vi "Preference_Panel.vi"(0 "Mode":T2) -> ()   [LabVIEW 2012]
uses:
  Anemometry Sub Vis/Controls/Server_Comms.ctl
  Anemometry Sub Vis/Controls/Preference_Mode.ctl
  Anemometry Sub Vis/Controls/EnFlo_Data_Folder_Setup.ctl
  Anemometry Sub Vis/File/Setup_Filetype.ctl
  Anemometry Sub Vis/Controls/Overhead.ctl
  <vilib>/Instr/_visa.llb/VISA Find Search Mode.ctl
  ADAM Client/Sub VIs/ADAM Controls/Ch_description_ADAM.ctl
  ADAM Client/Sub VIs/ADAM Controls/Module_type_ADAM.ctl
  ADAM Client/Sub VIs/ADAM Controls/Function_ADAM.ctl
  ADAM Client/Sub VIs/ADAM Controls/Channel_State.ctl
  ADAM Client/Sub VIs/ADAM Controls/Calib_type_ADAM.ctl
  ADAM Client/Sub VIs/ADAM Controls/Address.ctl
  Anemometry Sub Vis/Globals/Constants_global.vi
  Anemometry Sub Vis/Globals/Preference_global.vi
  Anemometry Sub Vis/Globals/Trav_pos_global.vi
  Anemometry Sub Vis/Acquisition/PWA/PWAtasksGLOBAL.vi
panel:
  in  "Traverse to Traverse Collision Detection":bool
  in  "DataTranslation Device No.":u32=20
  in  "Reset Email Counter":bool
  in  "EnFlo_Data_Folder_Setup":T1="EnFlo_Data on Server"
  in  "Post Processing Machine":bool
  in  "Analogue Device Serial No.":string="1188AB4"
  in  "PWA Device Serial No.":string="1187C98"
  in  "ADAM Setup File":u16(ring) items=["Scani_Valve.xls", "Current_Setup.xls"]
  in  "Default Source Establishment Time (s)":dbl=20.0
  out "This Machine's IP Number":string
  in  "Rig Setup":u16(ring) items=["3_x_2_tunnel", "A_Tunnel", "Adam_Sayer_Desk", "ADAM_Server", "Aero_Tunnel", "Alex_Desktop", "B_Tunnel", "Calibration_Tunnel", "Contact_Conductance", "D_Tunnel", "EnFlo_Tunnel", "Frauke_Desktop", "Fruit_Rig", "iMac_G5_2", "iMacDuo1", "Matteo's_desktop", "Matteo_PC", "Nick_PC-2", "Paul_Desk-Paul_Desk_Machine", "Paul_Hayden-Desk", "Paul_N_Desk_Machine_2", "phtest", "Post_Processing_Machine", "PowerBook_G4_1", "PowerBook_G4_2", "Syn_jet_rig", "Tank", "tdf", "Tom_Desk", "Towing_tank", "--New Rig Setup--"]
  in  "Default Traverse Name":u16(ring) items=["A_Tunnel", "Aero_Laser", "Aero_ThroughWall", "Aero_Tunnel", "Angle_Calibrator", "B_Tunnel", "D_Tunnel", "Dummy_Traverse", "EnFlo_Stack", "EnFlo_Tunnel", "EnFlo_Turntable", "Laser_Meas_Traverse", "mohd_setup", "Paul_Desk_Test", "PIV_Traverse", "--New Traverse Setup--"]
  in  "OK":bool
  in  "% Error From First Calib":dbl=10.0 format="%.1f"
  in  "% Error From Previous Calib":dbl=0.5 format="%.1f"
  out "Templates":path=path "/G4_2_HD/Applications (Mac OS 9)/EnFlo Software/Anemometry/Anemometry Sub Vis/Templates"
  in  "Data Folder":path
  out "EnFlo SW Preferences":path=path "/G4_2_HD/Applications (Mac OS 9)/LabVIEW 5.1/EnFlo SW Preferences"
  in  "Tunnel Speed Control":bool
  in  "SMTP server IP address":string
  in  "Abs Press (mbar)":string="Froude:NPL:Atmos_Press"
  in  "Temperature":string="EnFlo Tun:Inlet Heater:Av Temp"
  in  "Server port number":u32=3363
  in  "Server address":string
  in  "LabVIEW Administrators":string[](array[string])=["", "", "", "", "", "", "", "", "", "", "", "", "", "", "", "", "", "", "", ""]
  in  "Server Comms":T3=enum."Do Not Link To Server"
  # "Server Computer Peferences"
  # "Multi Run Preferences"
  # "Warning Levels for Autocalibration Changes"
  # "Email Peferences"
  # "Deg C"
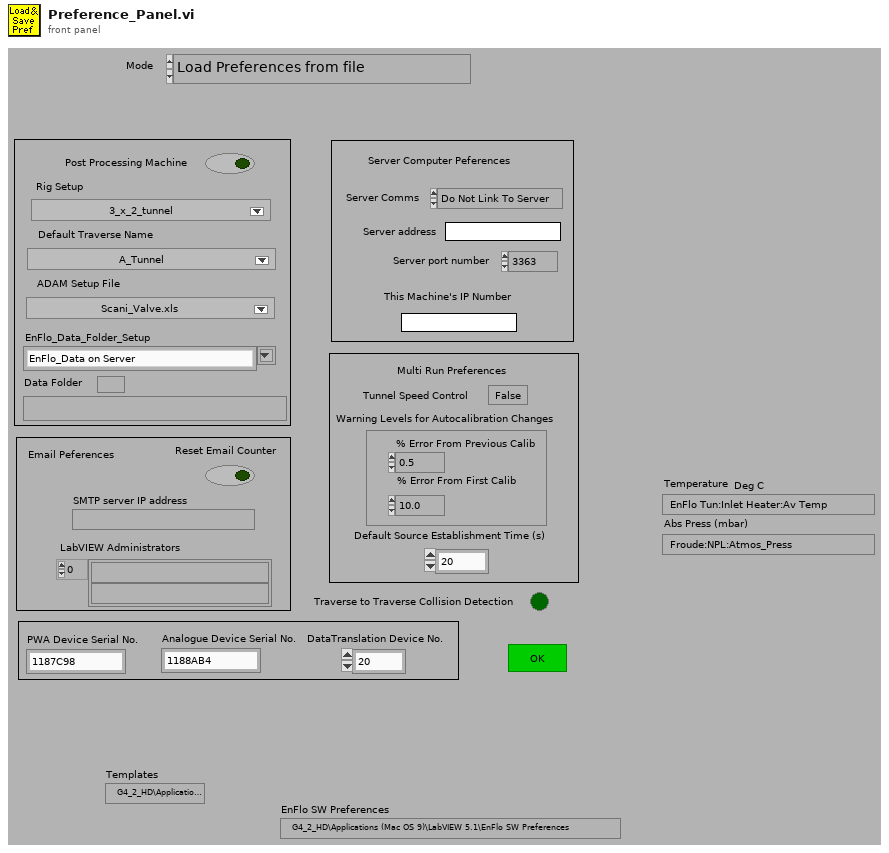
[diagram p1: front panel]
types:
  T1 = typedef "EnFlo_Data_Folder_Setup.ctl" = string
  T2 = typedef "Preference_Mode.ctl" = enum16{"Load Preferences from file", "Save Preferences to file", "Load, Edit then Save"}
  T3 = typedef "Server_Comms.ctl" = enum16{"Server Link Healthy", "Do Not Link To Server"}
  T4 = enum8{"Enabled", "Disabled", "Disabled and Grayed Out"}
  T5 = enum16{"Zero or one", "One", "Zero or more", "One or more"}
  T6 = typedef "Setup_Filetype.ctl" = enum16{"Measurement Setups", "Calibration Setups", "General", "Results File Plotter Setups", "Speed Calib Tweaks"}
  T7 = typedef "Overhead.ctl" = enum16{"Update total times", "Read Current Overhead", "Re Scale totals to 3 hrs", "Initialise totals to 3hr"}
  T8 = typedef "Calib_type_ADAM.ctl" = enum16{"Raw", "Bx + A", "Cx^2 + Bx + A", "Dx^3 + Cx^2 + Bx + A", "In Band", "Hi-Tec Q", "Hi-Tec M_dot", "Text"}
  T9 = typedef "Module_type_ADAM.ctl" = string
  T10 = typedef "Channel_State.ctl" = enum16{"On", "Off", "Always On", "Always Off"}
  T11 = typedef "LVDateTimeRec.ctl" = cluster{"fractional second":dbl, "second":i32, "minute":i32, "hour":i32, "day of month":i32, "month":i32, "year":i32, "day of week":i32, "day of year":i32, "DST":i32}
  T12 = typedef "VISA Find Search Mode.ctl" = u32
  T13 = typedef "Ch_description_ADAM.ctl" = cluster{"Ch Name":string, "Type":T9, "Function":T14, "Ch State":T10, "Calibration type":T8, "A":dbl, "B":dbl, "C":dbl, "D":dbl, "Comments":string, "Address":T15, "String":string, "Duty":u16}
  T14 = typedef "Function_ADAM.ctl" = enum16{"Analogue Input", "Digital Input", "Event counter", "Event rate", "Analogue Output", "Digital Output", "Relay Output"}
  T15 = typedef "Address.ctl" = cluster{"Main":i32, "Ch.":i32, "Sub":i32, "Port Name":string}
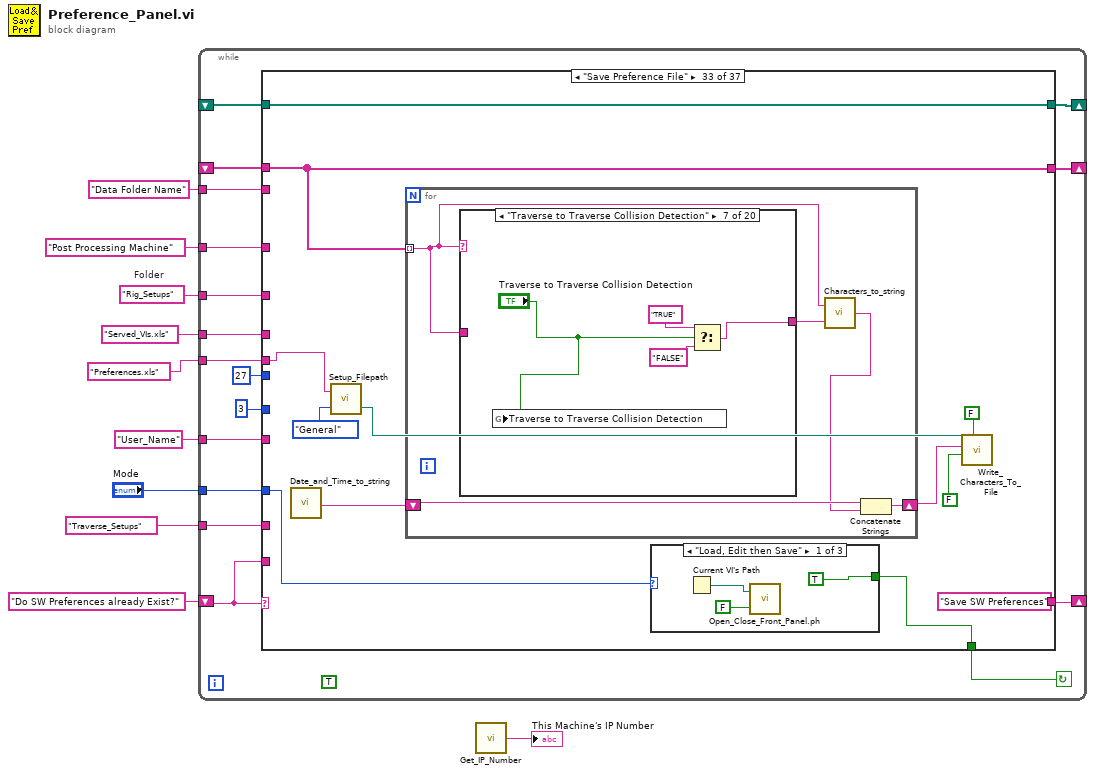
[diagram p0: block diagram]
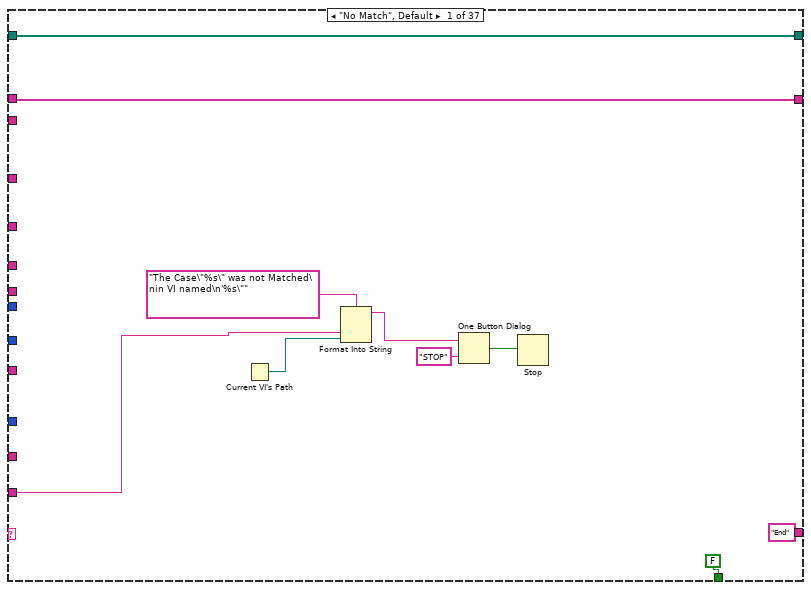
[diagram p2: hidden frame]
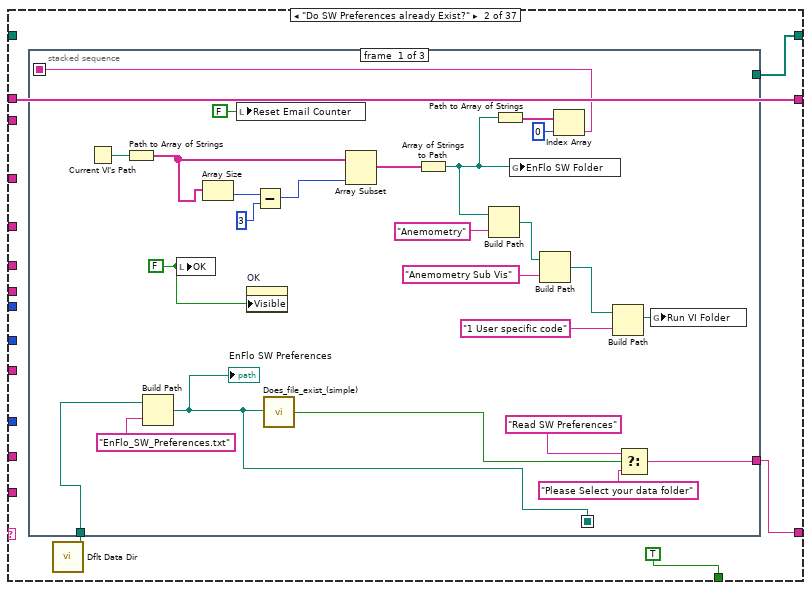
[diagram p3: hidden frame]
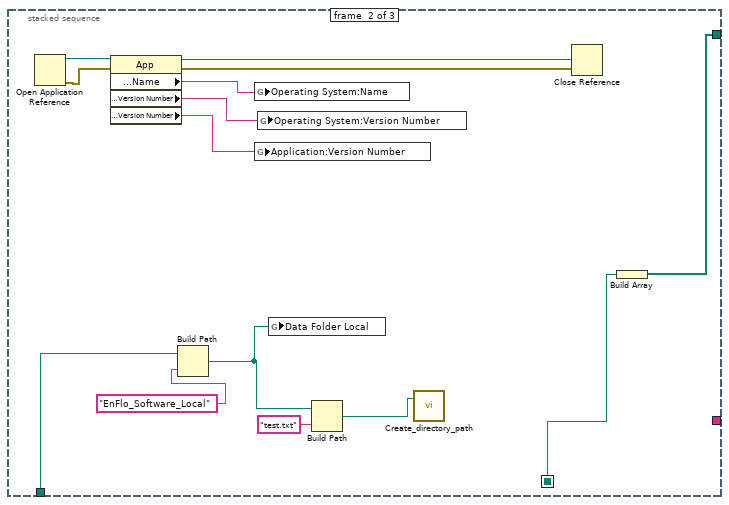
[diagram p4: hidden frame]
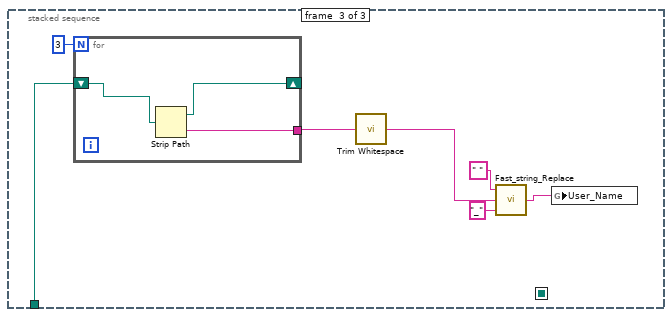
[diagram p5: hidden frame]
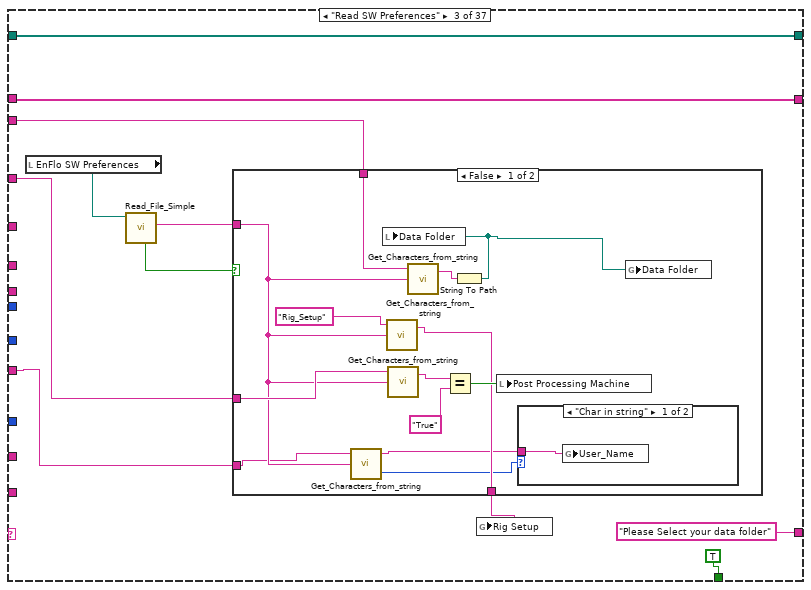
[diagram p6: hidden frame]
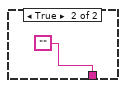
[diagram p8: hidden frame]
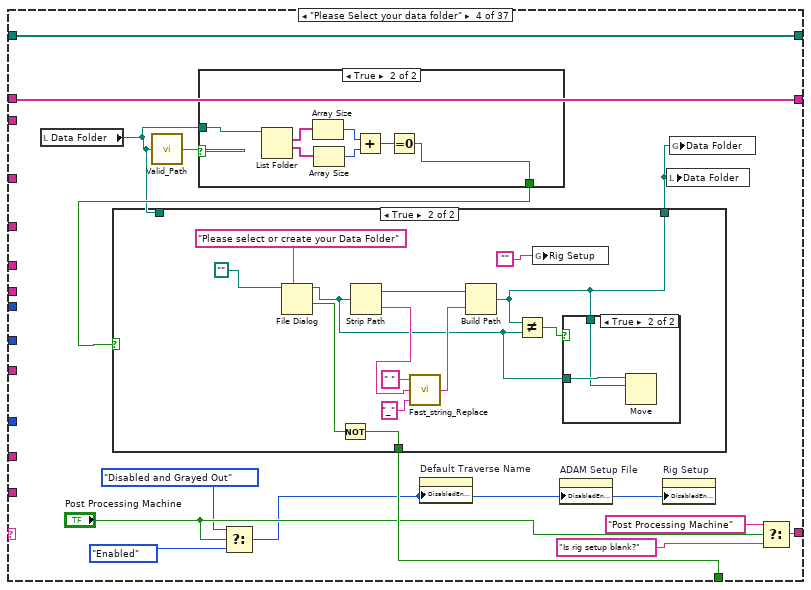
[diagram p9: hidden frame]
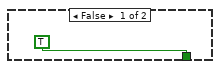
[diagram p10: hidden frame]
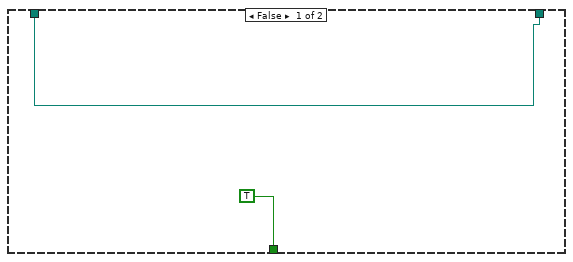
[diagram p11: hidden frame]
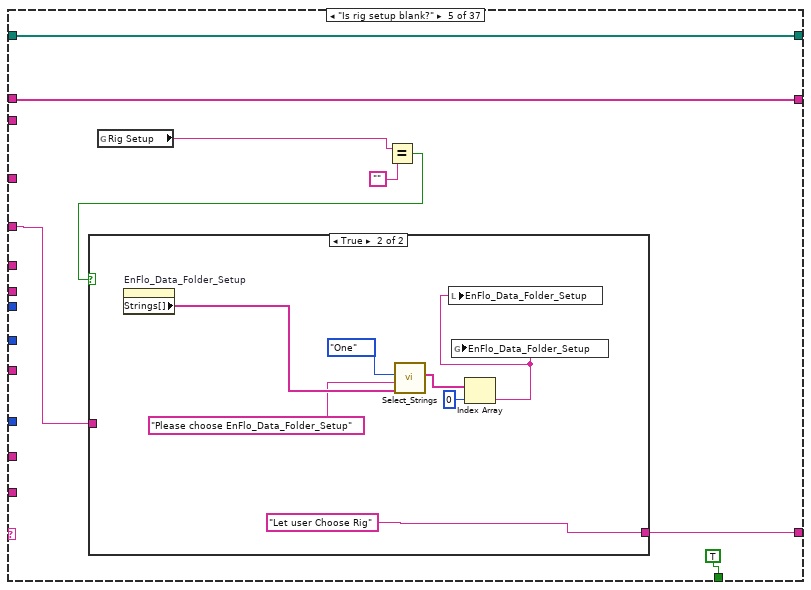
[diagram p13: hidden frame]
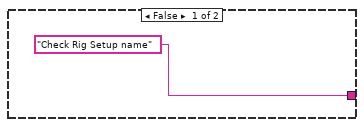
[diagram p14: hidden frame]
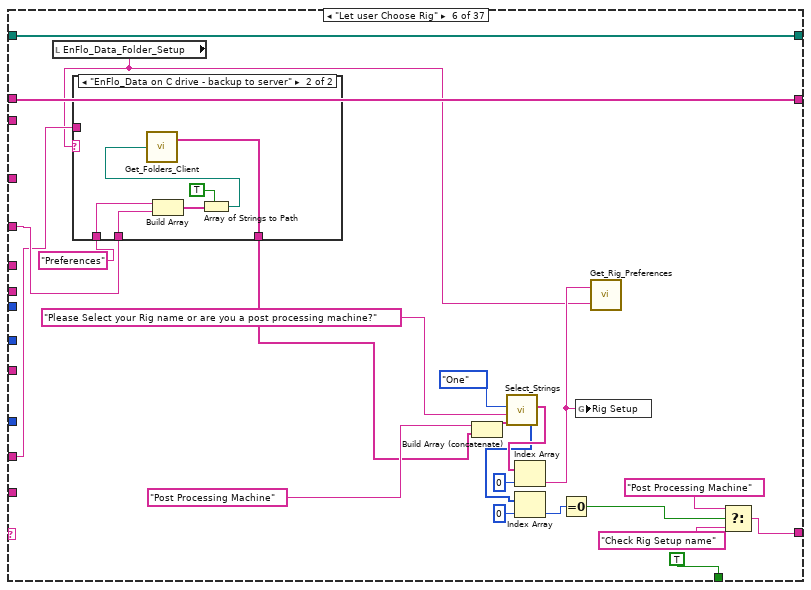
[diagram p15: hidden frame]
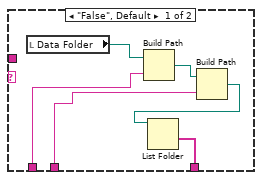
[diagram p16: hidden frame]
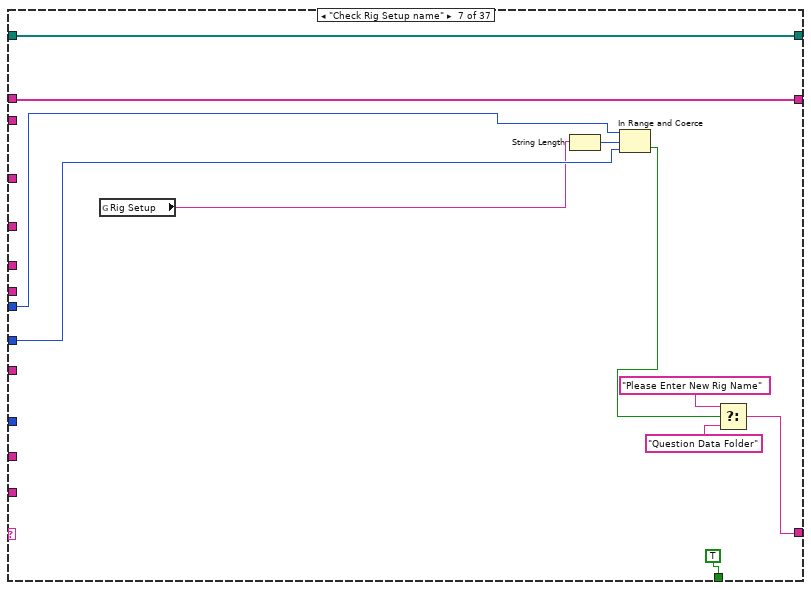
[diagram p17: hidden frame]
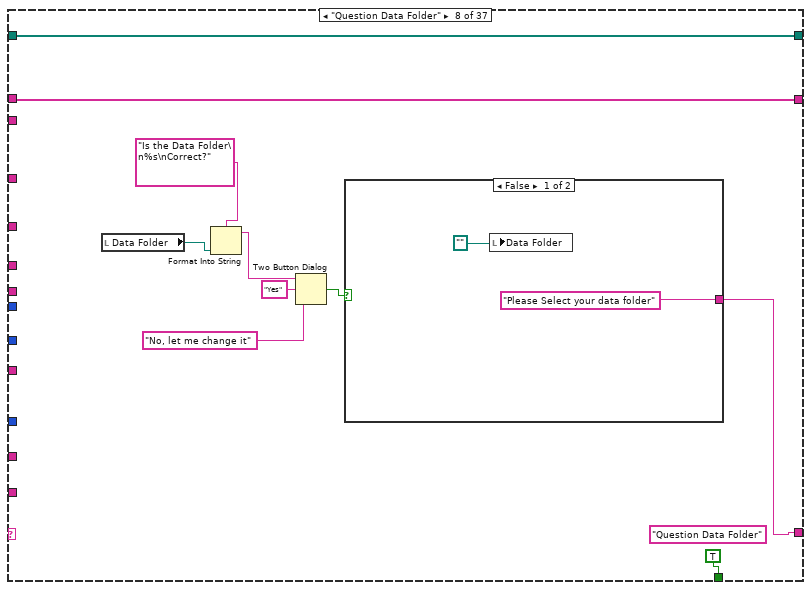
[diagram p18: hidden frame]
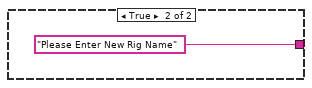
[diagram p19: hidden frame]
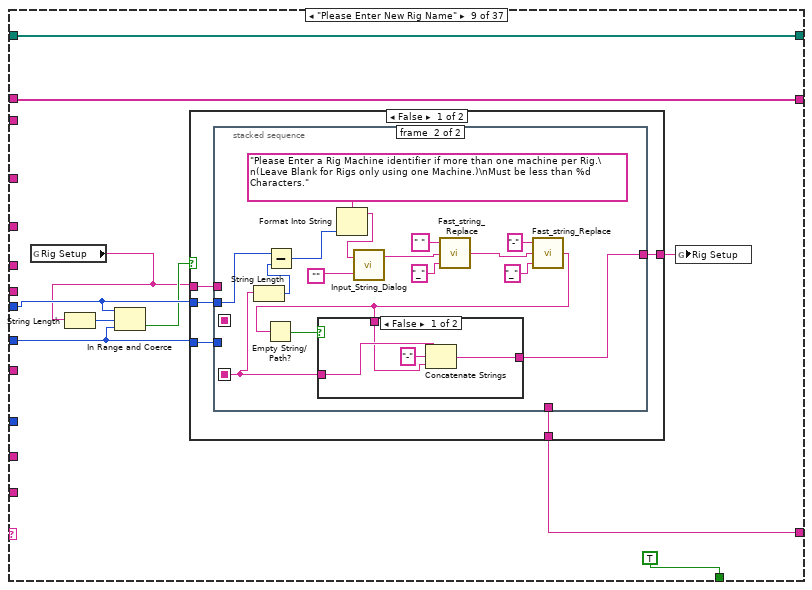
[diagram p20: hidden frame]
diagram:
  w5 = "Rig_Setups"  # Folder
  n1 = while {
    shift-left: _ -> [w24]
    shift-right: [w25] -> _
    shift-left: "Do SW Preferences already Exist?" -> [w12]
    shift-right: [w26] -> _
    tunnel: "Mode" -> [w23]
    tunnel: "Data Folder Name" ("Label for characters") -> [w22]
    tunnel: "Served_VIs.xls" ("Substring") -> [w21]
    tunnel: "Preferences.xls" ("name or relative path") -> [w20]
    tunnel: w5 -> [w17]
    tunnel: "Traverse_Setups" ("name or relative path") -> [w16]
    shift-right: [w15] -> _
    shift-left: _ -> [w14]
    tunnel: "Post Processing Machine" ("Label for characters") -> [w13]
    tunnel: "User_Name" ("Label for characters") -> [w11]
    stop <- w27 continue-if-true
    (unwired) TRUE ("append to file? (new file:F)")
    n2 = case shown="\"Save Preference File\"" w12 {
      tunnel: [FALSE TRUE TRUE w125 TRUE TRUE TRUE TRUE TRUE TRUE TRUE TRUE TRUE TRUE TRUE TRUE TRUE TRUE TRUE TRUE TRUE TRUE TRUE TRUE TRUE TRUE TRUE TRUE TRUE TRUE TRUE TRUE w924 TRUE TRUE TRUE FALSE] -> w27
      tunnel: ["End" w40 "Please Select your data folder" w122 w157 w190 w207 w218 w237 "Update Constants Global" ("f") "Copy Preferences?" "Copy Preferences?" w365 w375 "Install Preference files" "Install Adam table files" "Install Adam setup files" "Choose ADAM Setup file" "Preference files continued" "Variable Names" w553 w573 "Please Enter new  Traverse Setup" w652 "Create Traverse setup" ("f") "Check file permission status" w749 w780 w800 w820 w836 "Save Preference File" "Save SW Preferences" w999 w1013 "Initialise Globals" "End"] -> w26
      tunnel: [w29 w41 w101 w131 w163 w193 w216 w226 w239 w304 w330 w353 w363 w380 w438 w453 w478 w497 w519 w529 w558 w580 w640 w654 w688 w705 w750 w785 w805 w828 w841 w855 w930 w1007 w1014 w1066 w1125] -> w25
      tunnel: w24 -> [w29 w41 w101 w131 w163 w193 w216 w226 w239 w304 w330 w353 w363 w380 w438 w453 w478 w497 w519 w529 _ w580 w640 w654 w688 w705 w750 w785 w805 w828 w841 w855 w930 w1007 w1014 w1066 w1125]
      tunnel: w12 -> [w32 _ _ _ _ _ _ _ _ _ _ _ _ _ _ _ _ _ _ _ _ _ _ _ _ _ _ _ _ _ _ _ _ _ _ _ _]
      tunnel: w23 -> [_ _ _ _ _ _ _ _ _ _ _ _ _ _ _ _ _ _ _ _ w552 _ _ _ _ _ w748 _ _ _ _ _ w925 _ _ _ _]
      tunnel: w22 -> [_ _ w98 _ _ _ _ _ _ _ _ _ _ _ _ _ _ _ _ _ _ _ _ _ _ _ _ _ _ _ _ _ _ w998 _ _ _]
      tunnel: w21 -> [_ _ _ _ _ _ _ _ _ _ _ _ _ _ _ w448 _ _ _ _ _ _ _ _ _ _ _ _ _ _ _ _ _ _ _ w1058 _]
      tunnel: w20 -> [_ _ _ _ _ _ _ _ _ _ _ _ w359 w379 _ _ _ _ _ _ _ w570 _ _ _ _ _ _ _ _ _ _ w921 _ _ _ _]
      tunnel: 3 ("lower limit") -> [_ _ _ _ _ _ w212 _ w236 _ _ _ _ _ _ _ _ _ _ _ _ _ _ w651 _ _ _ _ _ _ _ _ _ _ _ _ _]
      tunnel: 27 ("upper limit") -> [_ _ _ _ _ _ w213 _ w235 _ _ _ _ _ _ _ _ _ _ _ _ _ _ w650 _ _ _ _ _ _ _ _ _ _ _ _ _]
      tunnel: w17 -> [_ _ _ _ w160 w178 _ _ _ w292 w318 _ _ w378 _ _ _ _ _ _ _ _ _ _ _ _ _ _ _ _ _ _ _ _ _ _ _]
      tunnel: w16 -> [_ _ _ _ _ w175 _ _ _ _ _ _ _ _ _ _ _ _ _ _ _ _ w638 _ w675 _ _ _ _ _ _ w854 _ _ _ _ _]
      tunnel: [w28 w38 w97 w126 w158 w192 w215 w225 w231 w290 w315 w342 w364 w381 w431 w444 w471 w494 w505 w521 w545 w576 w637 w646 w674 w701 path[] [] w777 w797 w823 w839 w853 w923 w995 w1012 w1060 w1123] -> w15
      tunnel: w14 -> [w28 _ w97 w126 w158 w192 w215 w225 w231 w290 w315 w342 w364 w381 w430 w446 w471 w495 w505 w523 w545 w577 w637 w646 w674 w702 w747 w777 w797 w823 w839 w853 w923 w995 w1012 w1060 w1123]
      tunnel: w13 -> [_ _ w96 _ _ _ _ _ _ _ _ _ _ _ _ _ _ _ _ _ _ _ _ _ _ _ _ _ _ _ _ _ _ w989 _ _ _]
      tunnel: w11 -> [_ _ w92 _ _ _ _ _ _ _ _ _ _ _ _ _ _ _ _ _ _ _ _ _ _ _ _ _ _ _ _ _ _ w988 _ _ _]
      frame "No Match", Default {
        n3 = Current VI's Path() -> (path=w37:path)
        n4 = Format Into String(format string="The Case\"%s\" was not Matched\nin VI named\n'%s\"" ("Format String"), w32, w37) -> (resulting string=w34:string)  [unwired: 2 in, 1 out]
        n5 = One Button Dialog(message=w34, button name ("OK")="STOP") -> (true=w36:bool)
        n6 = Stop(stop? (T)=w36) -> ()
      }
      frame "Do SW Preferences already Exist?" {
        n7 = call <vilib>:"Dflt Data Dir.vi"() -> ("App:Default Data Directory"=w39:path)
        n8 = stacked-sequence {
          seq-local: [w47 _ _] -> [_ _ _]
          seq-local: [w45 _ _] -> [_ w73 _]
          tunnel: [w51 _ _] -> w40
          tunnel: w39 -> [w46 w71 w87]
          tunnel: [_ w74 _] -> w38
          frame #0 {
            w44 = FALSE ("OK")
            n9 = Current VI's Path() -> (path=w65:path)
            n10 = Path to Array of Strings(0:w65) -> (2:w62:string[])  [unwired: 1 out]
            n11 = Build Path(base path=w46, name or relative path="EnFlo_SW_Preferences.txt") -> (appended path=w45:path)
            "EnFlo SW Preferences" <- w45
            n12 = local write "OK"(w44) -> ()
            n13 = Array Size(array=w62) -> (size(s)=w64:i32)
            n14 = local write "Reset Email Counter"(FALSE ("Reset Email Counter")) -> ()
            n15 = property on="OK" class="Bool (strict)"("Visible"=w44) -> ()  [unwired: 2 in, 2 out]
            n16 = Subtract(x=w64, y=3) -> (x-y=w60:i32)
            n17 = call "Does_file_exist_(simple).vi"("Pathname"=w45) -> ("exists?"=w66:bool)
            n18 = Array Subset(array=w62, length=w60) -> (w61:string[])  [unwired: 1 in]
            n19 = Array of Strings to Path(0:w61) -> (2:w48:path)  [unwired: 1 out]
            n20 = Build Path(base path=w48, name or relative path="Anemometry") -> (appended path=w57:path)
            n21 = Path to Array of Strings(0:w48) -> (2:w49:string[])  [unwired: 1 out]
            n22 = global write "Constants_global.vi" "EnFlo SW Folder"(w48) -> ()
            n23 = Build Path(base path=w57, name or relative path="Anemometry Sub Vis") -> (appended path=w55:path)
            n24 = Index Array(array=w49, index=0) -> (element=w47:string)
            n25 = Build Path(base path=w55, name or relative path="1 User specific code") -> (appended path=w54:path)
            n26 = Select(t="Read SW Preferences", s=w66, f="Please Select your data folder") -> (s? t:f=w51:string)
            n27 = global write "Constants_global.vi" "Run VI Folder"(w54) -> ()
          }
          frame #1 {
            n28 = Open Application Reference() -> (0:w78:errorcluster, 3:w81:refnum<vi>)  [unwired: 1 in, 3 out]
            n29 = property class="App"(reference=w81, error in=w78) -> (reference out=w80:refnum<vi>, error out=w79:errorcluster, "Operating System:Name"=w75:string, "Operating System:Version Number"=w77:string, "Application:Version Number"=w76:string)
            n30 = Build Path(base path=w71, name or relative path="EnFlo_Software_Local" ("element")) -> (appended path=w70:path)
            n31 = global write "Preference_global.vi" "Operating System:Name"(w75) -> ()
            n32 = global write "Preference_global.vi" "Application:Version Number"(w76) -> ()
            n33 = global write "Preference_global.vi" "Operating System:Version Number"(w77) -> ()
            n34 = global write "Constants_global.vi" "Data Folder Local"(w70) -> ()
            n35 = Build Path(base path=w70, name or relative path="test.txt") -> (appended path=w68:path)
            n36 = call "Create_directory_path.vi"("Path name"=w68) -> ()  [unwired: 1 in, 2 out]
            n37 = Close Reference(reference=w80, error in (no error)=w79) -> ()  [unwired: 1 out]
            n38 = Build Array(w73) -> (w74:path[])
          }
          frame #2 {
            n39 = for {
              N: 3 -> [_]
              shift-right: [w91] -> _
              shift-left: w87 -> [w90]
              tunnel: [w89] -> w83
              n40 = Strip Path(path=w90) -> (stripped path=w91:path, name=w89:string)
            }
            n41 = call <vilib>:"Trim Whitespace.vi"("string"=w83) -> ("trimmed string"=w82:string)  [unwired: 1 in]
            n42 = call "Fast_string_Replace.vi"("Replace match with:"="_", "Input String"=w82, "regular expression"=" ") -> ("Output String"=w84:string)  [unwired: 1 in, 1 out]
            n43 = global write "Preference_global.vi" "User_Name"(w84) -> ()
          }
        }
      }
      frame "Read SW Preferences" {
        n44 = local read "EnFlo SW Preferences"() -> (w100:path)
        n45 = call "Read_File_Simple.vi"("Filename"=w100) -> ("Error?"=w94:bool, "string"=w95:string)  [unwired: 2 in, 6 out]
        n46 = case shown="False" w94 {
          tunnel: w98 -> [w114 _]
          tunnel: w96 -> [w111 _]
          tunnel: w95 -> [w106 _]
          tunnel: [w107 ""] -> w93
          tunnel: w92 -> [w105 _]
          frame False {
            n47 = call "Get_Characters_from_string.vi"("Input string"=w106, "Variable name"=w105) -> ("Status"=w104:enum16{"Char in string", "Char not in string"}, "Value"=w103:string)  [unwired: 1 in]
            n48 = call "Get_Characters_from_string.vi"("Input string"=w106, "Variable name"="Rig_Setup" ("Label for characters")) -> ("Value"=w107:string)  [unwired: 1 in, 1 out]
            n49 = call "Get_Characters_from_string.vi"("Input string"=w106, "Variable name"=w111) -> ("Value"=w110:string)  [unwired: 1 in, 1 out]
            n50 = call "Get_Characters_from_string.vi"("Input string"=w106, "Variable name"=w114) -> ("Value"=w115:string)  [unwired: 1 in, 1 out]
            n51 = Equal?(x=w110, y="True") -> (x = y?=w108:bool)
            n52 = String To Path(string=w115) -> (path=w113:path)
            n53 = local write "Data Folder"(w113) -> ()
            n54 = local write "Post Processing Machine"(w108) -> ()
            n55 = case shown="\"Char in string\"" w104 {
              tunnel: w103 -> [w116 _]
              frame "Char in string" {
                n56 = global write "Preference_global.vi" "User_Name"(w116) -> ()
              }
              frame "Char not in string" {
              }
            }
            n57 = global write "Constants_global.vi" "Data Folder"(w113) -> ()
          }
          frame True {
          }
        }
        n58 = global write "Preference_global.vi" "Rig Setup"(w93) -> ()
      }
      frame "Please Select your data folder" {
        n59 = local read "Data Folder"() -> (w127:path)
        n60 = call "Valid_Path.vi"("Filename"=w127) -> ("Valid Path?"=w129:bool)
        n61 = case shown="True" w129 {
          tunnel: [TRUE ("status") w133] -> w128
          tunnel: w127 -> [_ w139]
          frame False {
          }
          frame True {
            n62 = List Folder(path=w139) -> (filenames=w137:string[], folder names=w138:string[])  [unwired: 1 in, 4 out]
            n63 = Array Size(array=w137) -> (size(s)=w135:i32)
            n64 = Array Size(array=w138) -> (size(s)=w136:i32)
            n65 = Add(x=w135, y=w136) -> (x+y=w134:i32)
            n66 = Equal To 0?(x=w134) -> (x = 0?=w133:bool)
          }
        }
        n67 = case shown="True" w128 {
          tunnel: [w141 w145] -> w130
          tunnel: w127 -> [w141 _]
          tunnel: [TRUE w143] -> w125
          frame False {
          }
          frame True {
            n68 = File Dialog(7:"Please select or create your Data Folder" ("prompt"), 11:path "") -> (1:w144:bool, 3:w146:path)  [unwired: 1 in, 6 out]
            n69 = Not(x=w144) -> (.not. x?=w143:bool)
            n70 = Strip Path(path=w146) -> (stripped path=w150:path, name=w149:string)
            n71 = call "Fast_string_Replace.vi"("Replace match with:"="_", "Input String"=w149, "regular expression"=" ") -> ("Output String"=w148:string)  [unwired: 2 out]
            n72 = Build Path(base path=w150, name or relative path=w148) -> (appended path=w145:path)
            n73 = Not Equal?(x=w145, y=w146) -> (x != y?=w147:bool)
            n74 = global write "Preference_global.vi" "Rig Setup"("") -> ()
            n75 = case shown="True" w147 {
              tunnel: w146 -> [_ w156]
              tunnel: w145 -> [_ w155]
              frame False {
              }
              frame True {
                n76 = Move(source path=w156, 10:w155) -> ()  [unwired: 1 in, 5 out]
              }
            }
          }
        }
        n77 = Select(t=T4."Disabled and Grayed Out" ("Disabled"), s="Post Processing Machine", f=T4."Enabled" ("Disabled")) -> (s? t:f=w118:T4)
        n78 = property on="Default Traverse Name" class="Ring (strict)"("DisabledEnum"=w118) -> ()  [unwired: 2 in, 2 out]
        n79 = property on="ADAM Setup File" class="Ring (strict)"("DisabledEnum"=w118) -> ()  [unwired: 2 in, 2 out]
        n80 = property on="Rig Setup" class="Ring (strict)"("DisabledEnum"=w118) -> ()  [unwired: 2 in, 2 out]
        n81 = local write "Data Folder"(w130) -> ()
        n82 = global write "Constants_global.vi" "Data Folder"(w130) -> ()
        n83 = Select(t="Post Processing Machine", s="Post Processing Machine", f="Is rig setup blank?") -> (s? t:f=w122:string)
      }
      frame "Is rig setup blank?" {
        n84 = global read "Preference_global.vi" "Rig Setup"() -> (w159:string)
        n85 = Equal?(x=w159, y="") -> (x = y?=w161:bool)
        n86 = case shown="True" w161 {
          tunnel: w160 -> [_ _]
          tunnel: ["Check Rig Setup name" ("t") "Let user Choose Rig"] -> w157
          frame False {
          }
          frame True {
            n87 = property on="EnFlo_Data_Folder_Setup" class="CmbBox (strict)"() -> ("Strings[]"=w170:string[])  [unwired: 2 in, 2 out]
            n88 = call "Select_Strings.vi"("Available Ch names"=w170, "Message"="Please choose EnFlo_Data_Folder_Setup", "Selector mode"=T5."One") -> ("Selected Channel Names"=w168:string[])  [unwired: 3 in, 2 out]
            n89 = Index Array(array=w168, index=0) -> (element=w166:string)
            n90 = local write "EnFlo_Data_Folder_Setup"(w166) -> ()
            n91 = global write "Preference_global.vi" "EnFlo_Data_Folder_Setup"(w166) -> ()
          }
        }
      }
      frame "Let user Choose Rig" {
        n92 = local read "EnFlo_Data_Folder_Setup"() -> (w173:T1)
        n93 = case shown="\"EnFlo_Data on C drive - backup to server\"" w173 {
          tunnel: "Preferences" ("name or relative path") -> [w198 w201]
          tunnel: w178 -> [w197 w206]
          tunnel: [w196 w203] -> w176
          tunnel: w175 -> [_ _]
          frame "False", Default {
            n94 = local read "Data Folder"() -> (w199:path)
            n95 = Build Path(base path=w199, name or relative path=w198) -> (appended path=w200:path)
            n96 = Build Path(base path=w200, name or relative path=w197) -> (appended path=w195:path)
            n97 = List Folder(path=w195) -> (folder names=w196:string[])  [unwired: 1 in, 5 out]
          }
          frame "EnFlo_Data on C drive - backup to server" {
            n98 = Build Array(w201, w206) -> (w205:string[])
            n99 = Array of Strings to Path(0:w205, 1:TRUE ("relative")) -> (2:w202:path)
            n100 = call "Get_Folders_Client.vi"("Relative Path"=w202) -> ("Folder Names"=w203:string[])  [unwired: 1 out]
          }
        }
        n101 = Build Array (concatenate)("Post Processing Machine", w176) -> (w183:string[])
        n102 = call "Select_Strings.vi"("Available Ch names"=w183, "Message"="Please Select your Rig name or are you a post processing machine?", "Selector mode"=T5."One") -> ("Ch Indicies Choosen"=w180:i32[], "Selected Channel Names"=w182:string[])  [unwired: 3 in, 1 out]
        n103 = Index Array(array=w182, index=0) -> (element=w174:string)
        n104 = Index Array(array=w180, index=0) -> (element=w179:i32)
        n105 = Equal To 0?(x=w179) -> (x = 0?=w189:bool)
        n106 = global write "Preference_global.vi" "Rig Setup"(w174) -> ()
        n107 = call "Get_Rig_Preferences.vi"("EnFlo_Data_Folder_Setup"=w173, "Rig Setup"=w174) -> ()  [unwired: 1 in]
        n108 = Select(t="Post Processing Machine", s=w189, f="Check Rig Setup name") -> (s? t:f=w190:string)
      }
      frame "Check Rig Setup name" {
        n109 = global read "Preference_global.vi" "Rig Setup"() -> (w208:string)
        n110 = String Length(string=w208) -> (length=w214:i32)
        n111 = In Range and Coerce(upper limit=w213, x=w214, lower limit=w212) -> (In Range?=w211:bool)  [unwired: 1 out]
        n112 = Select(t="Please Enter New Rig Name", s=w211, f="Question Data Folder") -> (s? t:f=w207:string)
      }
      frame "Question Data Folder" {
        (unwired) "Question Data Folder"
        n113 = local read "Data Folder"() -> (w224:path)
        n114 = Format Into String(format string="Is the Data Folder\n%s\nCorrect?" ("message"), w224) -> (resulting string=w222:string)  [unwired: 2 in, 1 out]
        n115 = Two Button Dialog(message=w222, 1:"No, let me change it" ("F button name (\"Cancel\")"), 2:"Yes" ("T button name (\"OK\")")) -> (T button?=w219:bool)
        n116 = case shown="False" w219 {
          tunnel: ["Please Select your data folder" "Please Enter New Rig Name"] -> w218
          frame False {
            n117 = local write "Data Folder"(path "") -> ()
          }
          frame True {
          }
        }
      }
      frame "Please Enter New Rig Name" {
        n118 = global read "Preference_global.vi" "Rig Setup"() -> (w233:string)
        n119 = String Length(string=w233) -> (length=w238:i32)
        n120 = In Range and Coerce(upper limit=w235, x=w238, lower limit=w236) -> (In Range?=w234:bool)  [unwired: 1 out]
        n121 = case shown="False" w234 {
          tunnel: w233 -> [w245 w288]
          tunnel: [w241 "Update Rig setup menu ring"] -> w237
          tunnel: [w242 w288] -> w232
          tunnel: w236 -> [w244 _]
          tunnel: w235 -> [w243 _]
          frame False {
            n122 = stacked-sequence {
              seq-local: [w246 _] -> [_ w271]
              seq-local: [w253 _] -> [_ _]
              tunnel: w245 -> [w255 _]
              tunnel: w244 -> [w266 _]
              tunnel: w243 -> [w252 w269]
              tunnel: [_ w274] -> w242
              tunnel: [w258 _] -> w241
              frame #0 {
                n123 = Match Pattern(string=w255, regular expression="-") -> (before substring=w254:string, after substring=w253:string)  [unwired: 3 out]
                n124 = String Length(string=w253) -> (length=w251:i32)
                n125 = Subtract(x=w252, y=w251) -> (x-y=w250:i32)
                n126 = Format Into String(format string="Please Enter a Rig Name.\n It must be between %d and %d Characters" ("Message to user"), w266, w250) -> (resulting string=w265:string)  [unwired: 2 in, 1 out]
                n127 = call "Input_String_Dialog.vi"("Value"=w254, "Message to user"=w265) -> ("Ok Out"=w261:bool, "Output string"=w262:string)
                n128 = call "Fast_string_Replace.vi"("Replace match with:"="_", "Input String"=w262, "regular expression"=" ") -> ("Output String"=w247:string)  [unwired: 2 out]
                n129 = Select(t="Please Enter New Rig Name", s=w261, f="Save Preference File") -> (s? t:f=w258:string)
                n130 = call "Fast_string_Replace.vi"("Replace match with:"="_", "Input String"=w247, "regular expression"="-") -> ("Output String"=w246:string)  [unwired: 2 out]
              }
              frame #1 {
                n131 = String Length(string=w271) -> (length=w270:i32)
                n132 = Subtract(x=w269, y=w270) -> (x-y=w268:i32)
                n133 = Format Into String(format string="Please Enter a Rig Machine identifier if more than one machine per Rig.\n(Leave Blank for Rigs only using one Machine.)\nMust be less than %d Characters." ("Message to user"), w268) -> (resulting string=w267:string)  [unwired: 2 in, 1 out]
                n134 = call "Input_String_Dialog.vi"("Value"="", "Message to user"=w267) -> ("Output string"=w280:string)  [unwired: 1 out]
                n135 = call "Fast_string_Replace.vi"("Replace match with:"="_", "Input String"=w280, "regular expression"=" ") -> ("Output String"=w276:string)  [unwired: 2 out]
                n136 = call "Fast_string_Replace.vi"("Replace match with:"="_", "Input String"=w276, "regular expression"="-") -> ("Output String"=w273:string)  [unwired: 2 out]
                n137 = Empty String/Path?(string/path=w273) -> (empty?=w275:bool)
                n138 = case shown="False" w275 {
                  tunnel: [w283 w287] -> w274
                  tunnel: w271 -> [w286 w287]
                  tunnel: w273 -> [w284 _]
                  frame False {
                    n139 = Concatenate Strings(w286, "-" ("string"), w284) -> (w283:string)
                  }
                  frame True {
                  }
                }
              }
            }
          }
          frame True {
          }
        }
        n140 = global write "Preference_global.vi" "Rig Setup"(w232) -> ()
      }
      frame "Update Rig setup menu ring" {
        n141 = local read "Data Folder"() -> (w295:path)
        n142 = Build Path(base path=w295, name or relative path="Preferences") -> (appended path=w294:path)
        n143 = global read "Preference_global.vi" "Rig Setup"() -> (w301:string)
        n144 = Build Path(base path=w294, name or relative path=w292) -> (appended path=w293:path)
        n145 = List Folder(path=w293) -> (folder names=w291:string[])  [unwired: 1 in, 5 out]
        n146 = Build Array (concatenate)(w291, "--New Rig Setup--") -> (w297:string[])
        n147 = Search 1D Array(1D array=w297, element=w301) -> (index of element=w300:i32)  [unwired: 1 out]
        n148 = case shown="-1" w300 {
          tunnel: [w307 0] -> w303
          tunnel: w297 -> [w306 w310]
          tunnel: w301 -> [_ w309]
          tunnel: w300 -> [w307 _]
          tunnel: [w306 w308] -> w299
          frame 0, Default {
          }
          frame -1 {
            n149 = Build Array (concatenate)(w309, w310) -> (w308:string[])
          }
        }
        n150 = local write "Rig Setup"(w303) -> ()
        n151 = property on="Rig Setup" class="Ring (strict)"("Strings []"=w299) -> ()  [unwired: 2 in, 2 out]
      }
      frame "Update Constants Global" {
        n152 = global read "Preference_global.vi" "Rig Setup"() -> (w317:string)
        n153 = global read "Constants_global.vi" "Data Folder"() -> (w316:path)
        n154 = Build Path(base path=w316, name or relative path="Preferences") -> (appended path=w319:path)
        n155 = Build Path(base path=w319, name or relative path=w318) -> (appended path=w320:path)
        n156 = Build Path(base path=w320, name or relative path=w317) -> (appended path=w312:path)
        n157 = Build Path(base path=w312, name or relative path="ADAM table") -> (appended path=w325:path)
        n158 = Build Path(base path=w312, name or relative path="Serial") -> (appended path=w324:path)
        n159 = Build Path(base path=w312, name or relative path="All_Users") -> (appended path=w313:path)
        n160 = Build Path(base path=w319, name or relative path="Traverse_Setups") -> (appended path=w323:path)
        n161 = global write "Constants_global.vi" "ADAM setups folder"(w325) -> ()
        n162 = global write "Constants_global.vi" "Serial setups folder"(w324) -> ()
        n163 = global write "Constants_global.vi" "All_Users"(w313) -> ()
        n164 = global write "Constants_global.vi" "Traverse folder"(w323) -> ()
        n165 = Build Array(w325, w324, w313, w323) -> (w322:path[])
        n166 = for {
          tunnel: w322 -> [w334] mode=indexing
          n167 = Build Path(base path=w334, name or relative path="Test") -> (appended path=w332:path)
          n168 = call "Create_directory_path.vi"("Path name"=w332) -> ()  [unwired: 1 in, 2 out]
        }
      }
      frame "Post Processing Machine" {
        n169 = global read "Constants_global.vi" "Data Folder Local"() -> (w341:path)
        n170 = global read "Preference_global.vi" "User_Name"() -> (w336:string)
        n171 = Build Path(base path=w341, name or relative path="Preferences") -> (appended path=w343:path)
        n172 = Build Path(base path=w343, name or relative path=w336) -> (appended path=w337:path)
        n173 = Build Path(base path=w337, name or relative path="ADAM table") -> (appended path=w348:path)
        n174 = Build Path(base path=w337, name or relative path="Serial") -> (appended path=w347:path)
        n175 = Build Path(base path=w337, name or relative path="All_Users") -> (appended path=w338:path)
        n176 = Build Path(base path=w343, name or relative path="Traverse_Setups") -> (appended path=w346:path)
        n177 = local write "Post Processing Machine"(TRUE ("Post Processing Machine")) -> ()
        n178 = global write "Constants_global.vi" "ADAM setups folder"(w348) -> ()
        n179 = global write "Constants_global.vi" "Serial setups folder"(w347) -> ()
        n180 = global write "Constants_global.vi" "All_Users"(w338) -> ()
        n181 = global write "Constants_global.vi" "Traverse folder"(w346) -> ()
        n182 = Build Array(w348, w347, w338, w346) -> (w345:path[])
        n183 = for {
          tunnel: w345 -> [w357] mode=indexing
          n184 = Build Path(base path=w357, name or relative path="Test") -> (appended path=w355:path)
          n185 = call "Create_directory_path.vi"("Path name"=w355) -> ()  [unwired: 1 in, 2 out]
        }
        n186 = global write "Preference_global.vi" "Rig Setup"("Post_Processing_Machine" ("Rig Setup")) -> ()
      }
      frame "Copy Preferences?" {
        n187 = call "Setup_Filepath.vi"("Setup File Type"=Setup_Filetype."General", "Filename in"=w359) -> ("Filename Out"=w358:path)  [unwired: 1 out]
        n188 = call <vilib>:"Check if File or Folder Exists.vi"("path"=w358) -> ("file or folder exists?"=w362:bool)  [unwired: 1 in, 9 out]
        n189 = case shown="False" w362 {
          tunnel: [w369 TRUE ("Error?")] -> w361
          frame False {
            n190 = global read "Constants_global.vi" "All_Users"() -> (w371:path)
            n191 = Build Path(base path=w371, name or relative path="Current_Username") -> (appended path=w372:path)
            n192 = call "Read_File_Simple.vi"("Filename"=w372) -> ("Error?"=w369:bool)  [unwired: 4 in, 5 out]
          }
          frame True {
          }
        }
        n193 = Select(t="Install Generic Meas Setup file", s=w361, f="Copy from last user") -> (s? t:f=w365:string)
      }
      frame "Copy from last user" {
        n194 = stacked-sequence {
          seq-local: [w392 _ _ _] -> [_ w402 w411 w423]
          seq-local: [_ w397 _ _] -> [_ _ _ w417]
          seq-local: [_ _ w406 _] -> [_ _ _ w416]
          tunnel: w379 -> [_ w400 _ _]
          tunnel: w378 -> [_ _ _ _]
          tunnel: [_ _ _ w415] -> w377
          frame #0 {
            n195 = global read "Constants_global.vi" "All_Users"() -> (w396:path)
            n196 = Seconds To Date/Time() -> (date time rec=w387:T11)  [unwired: 2 out]
            n197 = Unbundle By Name(w387) -> ("year"=w388:i32)
            n198 = global read "Preference_global.vi" "Rig Setup"() -> (w385:string)
            n199 = Build Path(base path=w396, name or relative path="Current_Username") -> (appended path=w394:path)
            n200 = Number To Decimal String(number=w388) -> (decimal integer string=w386:string)  [unwired: 1 out]
            n201 = global read "Constants_global.vi" "Data Folder"() -> (w391:path)
            n202 = call "Read_File_Simple.vi"("Filename"=w394) -> ("string"=w384:string)  [unwired: 4 in, 5 out]
            n203 = Build Path(base path=w391, name or relative path=w386) -> (appended path=w390:path)
            n204 = Build Path(base path=w390, name or relative path=w385) -> (appended path=w389:path)
            n205 = Build Path(base path=w389, name or relative path=w384) -> (appended path=w393:path)
            n206 = Build Path(base path=w393, name or relative path="Preferences") -> (appended path=w392:path)
          }
          frame #1 {
            n207 = call "Setup_Filepath.vi"("Setup File Type"=Setup_Filetype."General", "Filename in"=w400) -> ("Filename Out"=w399:path)  [unwired: 1 out]
            n208 = Build Path(base path=w402, name or relative path="General") -> (appended path=w404:path)
            n209 = Build Path(base path=w404, name or relative path=w400) -> (appended path=w403:path)
            n210 = Copy(10:w399, 11:w403) -> (0:w398:errorcluster)  [unwired: 3 in, 2 out]
            n211 = Unbundle By Name(w398) -> ("status"=w397:bool)
          }
          frame #2 {
            w409 = "Current_Setup.xls"
            n212 = Build Path(base path=w411, name or relative path="Meas Setups") -> (appended path=w413:path)
            n213 = Build Path(base path=w413, name or relative path=w409) -> (appended path=w412:path)
            n214 = call "Setup_Filepath.vi"("Setup File Type"=Setup_Filetype."Measurement Setups", "Filename in"=w409) -> ("Filename Out"=w408:path)  [unwired: 1 out]
            n215 = Copy(10:w408, 11:w412) -> (0:w407:errorcluster)  [unwired: 3 in, 2 out]
            n216 = Unbundle By Name(w407) -> ("status"=w406:bool)
          }
          frame #3 {
            w421 = "Current_Setup.xls"
            n217 = Build Path(base path=w423, name or relative path="Calib Setups") -> (appended path=w425:path)
            n218 = Build Path(base path=w425, name or relative path=w421) -> (appended path=w424:path)
            n219 = call "Setup_Filepath.vi"("Setup File Type"=Setup_Filetype."Calibration Setups", "Filename in"=w421) -> ("Filename Out"=w420:path)  [unwired: 1 out]
            n220 = Copy(10:w420, 11:w424) -> (0:w419:errorcluster)  [unwired: 3 in, 2 out]
            n221 = Unbundle By Name(w419) -> ("status"=w418:bool)
            n222 = Compound Arithmetic op=OR(w418, w417, w416) -> (w415:bool)
          }
        }
        n223 = Select(t="Install Generic Meas Setup file", s=w377, f="Read SW Preferences") -> (s? t:f=w375:string)
      }
      frame "Install Generic Meas Setup file" {
        n224 = global read "Constants_global.vi" "Run VI Folder"() -> (w437:path)
        n225 = Strip Path(path=w437) -> (stripped path=w435:path)  [unwired: 1 out]
        n226 = call "Setup_Filepath.vi"("Setup File Type"=Setup_Filetype."Measurement Setups", "Filename in"="Current_Setup.xls" ("name or relative path")) -> ("Filename Out"=w427:path)  [unwired: 1 out]
        n227 = Build Path(base path=w435, name or relative path="Templates") -> (appended path=w433:path)
        "Templates" <- w433
        n228 = call "Does_file_exist_(simple).vi"("Pathname"=w427) -> ("exists?"=w434:bool)
        n229 = case shown="False" w434 {
          tunnel: w427 -> [w443 _]
          tunnel: w433 -> [w441 _]
          frame False {
            n230 = Build Path(base path=w441, name or relative path="Measurement Setup.xls") -> (appended path=w440:path)
            n231 = Copy(10:w443, 11:w440) -> ()  [unwired: 1 in, 5 out]
          }
          frame True {
          }
        }
        n232 = Build Array (concatenate)(w430, w427) -> (w431:path[])
      }
      frame "Install Preference files" {
        n233 = Build Array("Preferences.xls" ("Substring"), w448, "Month_Names.xls" ("name or relative path"), "LDA_Configuration.xls") -> (w452:string[])
        n234 = for {
          tunnel: w452 -> [w456] mode=indexing
          tunnel: [w455] -> w445 mode=indexing
          n235 = call "Setup_Filepath.vi"("Setup File Type"=Setup_Filetype."General", "Filename in"=w456) -> ("Filename Out"=w455:path)  [unwired: 1 out]
          n236 = call "Does_file_exist_(simple).vi"("Pathname"=w455) -> ("exists?"=w458:bool)
          n237 = case shown="False" w458 {
            tunnel: w455 -> [w462 _]
            tunnel: w456 -> [w459 _]
            frame False {
              n238 = local read "Templates"() -> (w460:path)
              n239 = Build Path(base path=w460, name or relative path=w459) -> (appended path=w461:path)
              n240 = Copy(10:w462, 11:w461) -> ()  [unwired: 1 in, 5 out]
            }
            frame True {
            }
          }
        }
        n241 = Build Array (concatenate)(w446, w445) -> (w444:path[])
      }
      frame "Install Adam table files" {
        w467 = "Current_Setup.xls"
        n242 = global read "Constants_global.vi" "ADAM setups folder"() -> (w469:path)
        n243 = Build Path(base path=w469, name or relative path=w467) -> (appended path=w470:path)
        n244 = Build Path(base path=w469, name or relative path="Setup_Files") -> (appended path=w465:path)
        n245 = Build Array("Hi_Tec_Calibs.xls" ("name or relative path"), "A_Tunnel DB setup.xls" ("Substring"), "EnFlo_Tunnel DB setup.xls", "Aero_Tunnel DB setup.xls" ("name or relative path"), "D_Tunnel DB setup.xls") -> (w477:string[])
        n246 = Build Path(base path=w465, name or relative path=w467) -> (appended path=w464:path)
        n247 = for {
          tunnel: w477 -> [w481] mode=indexing
          tunnel: w469 -> [w482]
          n248 = Build Path(base path=w482, name or relative path=w481) -> (appended path=w480:path)
          n249 = call "Does_file_exist_(simple).vi"("Pathname"=w480) -> ("exists?"=w483:bool)
          n250 = case shown="False" w483 {
            tunnel: w480 -> [w487 _]
            tunnel: w481 -> [w484 _]
            frame False {
              n251 = local read "Templates"() -> (w485:path)
              n252 = Build Path(base path=w485, name or relative path=w484) -> (appended path=w486:path)
              n253 = Copy(10:w487, 11:w486) -> ()  [unwired: 1 in, 5 out]
            }
            frame True {
            }
          }
        }
        n254 = call "Create_directory_path.vi"("Path name"=w464) -> ("Path name Out"=w463:path)  [unwired: 1 in, 1 out]
        n255 = Move(source path=w470, 10:w463) -> ()  [unwired: 1 in, 5 out]
      }
      frame "Install Adam setup files" {
        w491 = "Current_Setup.xls"
        n256 = global read "Constants_global.vi" "ADAM setups folder"() -> (w493:path)
        n257 = Build Path(base path=w493, name or relative path="Setup_Files") -> (appended path=w490:path)
        n258 = Build Path(base path=w490, name or relative path=w491) -> (appended path=w488:path)
        n259 = call "Does_file_exist_(simple).vi"("Pathname"=w488) -> ("exists?"=w489:bool)
        n260 = case shown="False" w489 {
          tunnel: w488 -> [w504 _]
          tunnel: w491 -> [w502 _]
          frame False {
            n261 = local read "Templates"() -> (w503:path)
            n262 = Build Path(base path=w503, name or relative path="ADAM_Setup_files") -> (appended path=w501:path)
            n263 = Build Path(base path=w501, name or relative path=w502) -> (appended path=w500:path)
            n264 = Copy(10:w504, 11:w500) -> ()  [unwired: 1 in, 5 out]
          }
          frame True {
          }
        }
        n265 = Build Array (concatenate)(w495, w488) -> (w494:path[])
      }
      frame "Choose ADAM Setup file" {
        w513 = "Selected_Filename.txt" ("Substring")
        n266 = global read "Constants_global.vi" "ADAM setups folder"() -> (w517:path)
        n267 = Build Path(base path=w517, name or relative path="Setup_Files") -> (appended path=w514:path)
        n268 = Build Path(base path=w514, name or relative path=w513) -> (appended path=w512:path)
        n269 = call "Read_File_Simple.vi"("Filename"=w512) -> ("string"=w510:string)  [unwired: 2 in, 7 out]
        n270 = Build Array(w513) -> (w515:string[])
        n271 = call "List_files_in_order_of_age.vi"("Files to Hide"=w515, "Folder"=w514) -> ("file names"=w511:string[])
        n272 = Search 1D Array(1D array=w511, element=w510) -> (index of element=w507:i32)  [unwired: 1 out]
        n273 = property on="ADAM Setup File" class="Ring (strict)"("Strings []"=w511) -> ()  [unwired: 2 in, 2 out]
        n274 = Less Than 0?(x=w507) -> (x < 0?=w508:bool)
        n275 = Select(t=0, s=w508, f=w507) -> (s? t:f=w506:i32)
        n276 = local write "ADAM Setup File"(w506) -> ()
      }
      frame "Preference files continued" {
        n277 = Build Array("Hot_Wire_Bridges.txt", "Hot_Wire_Probes.txt", "Pressure_Transducers.txt") -> (w524:string[])
        n278 = for {
          tunnel: w524 -> [w532] mode=indexing
          tunnel: [w531] -> w522 mode=indexing
          n279 = call "Setup_Filepath.vi"("Setup File Type"=Setup_Filetype."Calibration Setups", "Filename in"=w532) -> ("Filename Out"=w531:path)  [unwired: 1 out]
          n280 = call "Does_file_exist_(simple).vi"("Pathname"=w531) -> ("exists?"=w534:bool)
          n281 = case shown="False" w534 {
            tunnel: w531 -> [w538 _]
            tunnel: w532 -> [w535 _]
            frame False {
              n282 = local read "Templates"() -> (w536:path)
              n283 = Build Path(base path=w536, name or relative path=w535) -> (appended path=w537:path)
              n284 = Copy(10:w538, 11:w537) -> ()  [unwired: 1 in, 5 out]
            }
            frame True {
            }
          }
        }
        n285 = Build Array (concatenate)(w523, w522) -> (w521:path[])
      }
      frame "Variable Names" {
        n286 = Build Array("Traverse to Traverse Collision Detection", "DataTranslation Device No.", "PWA Device Serial No.", "Analogue Device Serial No.", "Server address", "Server port number", "LabVIEW Administrators", "SMTP server IP address", "Server Comms", "Default Source Establishment Time (s)", "Temperature", "Abs Press (mbar)", "Default Traverse Name", "Tunnel Speed Control", "Current Overhead Factor", "EnFlo_Data_Central_Repository", "Auto Calib Error fr Previous", "Auto Calib Error fr First", "EnFlo_Data_Folder_Setup") -> (w558:string[])
        n287 = case shown="\"Load, Edit then Save\"" w552 {
          tunnel: ["Load From Preference file" w564 "Save Preference File"] -> w553
          frame "Load Preferences from file" {
          }
          frame "Load, Edit then Save" {
            n288 = local read "OK"() -> (w567:bool)
            n289 = Select(t="Save Preference File", s=w567, f="Load From Preference file") -> (s? t:f=w564:string)
          }
          frame "Save Preferences to file" {
          }
        }
      }
      frame "Load From Preference file" {
        n290 = call "Setup_Filepath.vi"("Setup File Type"=Setup_Filetype."General", "Filename in"=w570) -> ("Filename Out"=w569:path)  [unwired: 1 out]
        n291 = call "Read_File_Simple.vi"("Filename"=w569) -> ("string"=w578:string)  [unwired: 2 in, 7 out]
        n292 = for {
          tunnel: w580 -> [w583] mode=indexing
          tunnel: w578 -> [w582]
          w585 = FALSE  # Show Dialog?
          n293 = call "Get_Characters_from_string.vi"("Show Dialog?"=w585, "Input string"=w582, "Variable name"=w583) -> ("Status"=w584:enum16{"Char in string", "Char not in string"}, "Value"=w581:string)
          n294 = case shown="\"Char in string\"" w584 {
            tunnel: w583 -> [w587 _]
            tunnel: w581 -> [w586 _]
            frame "Char in string" {
              n295 = case shown="\"Traverse to Traverse Collision Detection\"" w587 {
                tunnel: w587 -> [w589 _ _ _ _ _ _ _ _ _ _ _ _ _ _ _ _ _ _ _]
                tunnel: w586 -> [_ w590 w591 w594 w595 w598 w599 w600 w602 w604 w607 w610 _ w614 w618 w619 w621 w623 w626 w628]
                tunnel: w586 -> [_ _ _ _ _ _ _ _ _ _ _ _ w611 _ _ _ _ _ _ _]
                frame "No Match", Default {
                  n296 = call "Was_string_matched.vi"("Match Error"=TRUE, "Variable name"=w589) -> ()  [unwired: 1 in]
                }
                frame "Server address" {
                  n297 = global write "Preference_global.vi" "Server address"(w590) -> ()
                  n298 = local write "Server address"(w590) -> ()
                }
                frame "EnFlo_Data_Folder_Setup" {
                  n299 = local write "EnFlo_Data_Folder_Setup"(w591) -> ()
                  n300 = global write "Preference_global.vi" "EnFlo_Data_Folder_Setup"(w591) -> ()
                }
                frame "DataTranslation Device No." {
                  n301 = Decimal String To Number(string=w594, default (0L)=u32 0 ("default (0 I32)")) -> (number=w592:u32)  [unwired: 1 in, 1 out]
                  n302 = global write "Preference_global.vi" "DataTranslation Device No."(w592) -> ()
                  n303 = local write "DataTranslation Device No."(w592) -> ()
                }
                frame "Default Traverse Name" {
                  n304 = global write "Trav_pos_global.vi" "Default Traverse Setup"(w595) -> ()
                }
                frame "Server port number" {
                  n305 = Decimal String To Number(string=w598) -> (number=w597:i32)  [unwired: 3 out]
                  n306 = To Unsigned Long Integer(number=w597) -> (unsigned 32bit integer=w596:u32)
                  n307 = local write "Server port number"(w596) -> ()
                  n308 = global write "Preference_global.vi" "Server port number"(w596) -> ()
                }
                frame "Analogue Device Serial No." {
                  n309 = local write "Analogue Device Serial No."(w599) -> ()
                }
                frame "PWA Device Serial No." {
                  n310 = local write "PWA Device Serial No."(w600) -> ()
                }
                frame "Default Source Establishment Time (s)" {
                  n311 = Fract/Exp String To Number(string=w602) -> (number=w601:dbl)  [unwired: 4 out]
                  n312 = global write "Preference_global.vi" "Default Source Establishment Time (s)"(w601) -> ()
                  n313 = local write "Default Source Establishment Time (s)"(w601) -> ()
                }
                frame "Tunnel Speed Control" {
                  n314 = Equal?(x="TRUE", y=w604) -> (x = y?=w603:bool)
                  n315 = local write "Tunnel Speed Control"(w603) -> ()
                  n316 = global write "Preference_global.vi" "Tunnel Speed Control"(w603) -> ()
                }
                frame "Traverse to Traverse Collision Detection" {
                  n317 = Equal?(x="TRUE", y=w607) -> (x = y?=w606:bool)
                  n318 = global write "Preference_global.vi" "Traverse to Traverse Collision Detection"(w606) -> ()
                  n319 = local write "Traverse to Traverse Collision Detection"(w606) -> ()
                }
                frame "LabVIEW Administrators" {
                  n320 = call "Get_array_values_fr_String.vi"("String Value"=w610) -> ("String array"=w609:string[])  [unwired: 1 out]
                  n321 = global write "Preference_global.vi" "LabVIEW Administrators"(w609) -> ()
                  n322 = local write "LabVIEW Administrators"(w609) -> ()
                }
                frame "SMTP server IP address" {
                  n323 = local write "SMTP server IP address"(w611) -> ()
                  n324 = global write "Preference_global.vi" "SMTP server IP address"(w611) -> ()
                }
                frame "Server Comms" {
                  n325 = Equal?(x="TRUE", y=w614) -> (x = y?=w613:bool)
                  n326 = case shown="False" w613 {
                    tunnel: [Server_Comms."Do Not Link To Server" ("Server Comms") Server_Comms."Server Link Healthy" ("Server Comms")] -> w612
                    frame False {
                    }
                    frame True {
                    }
                  }
                  n327 = local write "Server Comms"(w612) -> ()
                  n328 = global write "Preference_global.vi" "Server Comms"(w612) -> ()
                }
                frame "Temperature" {
                  n329 = global write "Preference_global.vi" "Temperature"(w618) -> ()
                  n330 = local write "Temperature"(w618) -> ()
                }
                frame "Abs Press (mbar)" {
                  n331 = global write "Preference_global.vi" "Abs Press (mbar)"(w619) -> ()
                  n332 = local write "Abs Press (mbar)"(w619) -> ()
                }
                frame "EnFlo_Data_Central_Repository" {
                  n333 = String To Path(string=w621) -> (path=w620:path)
                  n334 = global write "Constants_global.vi" "EnFlo_Data_Central_Repository"(w620) -> ()
                }
                frame "Current Overhead Factor" {
                  n335 = Fract/Exp String To Number(string=w623) -> (number=w622:dbl)  [unwired: 4 out]
                  n336 = call "Overhead_Factor.vi"("Current Overhead Factor In"=w622, "Mode"=Overhead."Initialise totals to 3hr") -> ()  [unwired: 2 in, 1 out]
                }
                frame "Auto Calib Error fr Previous" {
                  n337 = Fract/Exp String To Number(string=w626) -> (number=w625:dbl)  [unwired: 4 out]
                  n338 = global write "Preference_global.vi" "% Error From Previous Calib"(w625) -> ()
                  n339 = local write "% Error From Previous Calib"(w625) -> ()
                }
                frame "Auto Calib Error fr First" {
                  n340 = Fract/Exp String To Number(string=w628) -> (number=w627:dbl)  [unwired: 4 out]
                  n341 = global write "Preference_global.vi" "% Error From First Calib"(w627) -> ()
                  n342 = local write "% Error From First Calib"(w627) -> ()
                }
              }
            }
            frame "Char not in string" {
            }
          }
        }
        n343 = local read "Post Processing Machine"() -> (w575:bool)
        n344 = Select(t="Check file permission status", s=w575, f="is traverse setup blank?") -> (s? t:f=w573:string)
        n345 = Build Array (concatenate)(w577, w569) -> (w576:path[])
      }
      frame "is traverse setup blank?" {
        n346 = local read "Data Folder"() -> (w635:path)
        n347 = global read "Trav_pos_global.vi" "Default Traverse Setup"() -> (w629:string)
        n348 = Build Path(base path=w635, name or relative path="Preferences") -> (appended path=w634:path)
        n349 = Build Path(base path=w634, name or relative path=w638) -> (appended path=w633:path)
        n350 = List Folder(path=w633) -> (folder names=w631:string[])  [unwired: 1 in, 5 out]
        n351 = Search 1D Array(1D array=w631, element=w629) -> (index of element=w632:i32)  [unwired: 1 out]
        n352 = case shown="0, Default" w632 {
          tunnel: w631 -> [_ w644]
          tunnel: [w642 w643] -> w630
          tunnel: w629 -> [w642 _]
          frame 0, Default {
          }
          frame -1 {
            n353 = Index Array(array=w644, index=0) -> (element=w643:string)
          }
        }
        n354 = global write "Trav_pos_global.vi" "Default Traverse Setup"(w630) -> ()
      }
      frame "Please Enter new  Traverse Setup" {
        n355 = global read "Trav_pos_global.vi" "Default Traverse Setup"() -> (w648:string)
        n356 = String Length(string=w648) -> (length=w653:i32)
        n357 = In Range and Coerce(upper limit=w650, x=w653, lower limit=w651) -> (In Range?=w649:bool)  [unwired: 1 out]
        n358 = case shown="False" w649 {
          tunnel: w648 -> [w664 w672]
          tunnel: ["Please Enter new  Traverse Setup" "Update Traverse setup menu ring"] -> w652
          tunnel: [w657 w672] -> w647
          tunnel: w651 -> [w661 _]
          tunnel: w650 -> [w660 _]
          frame False {
            n359 = Format Into String(format string="Please Enter a Traverse Setup Name\nIt must be between %d and %d Characters" ("Message to user"), w661, w660) -> (resulting string=w659:string)  [unwired: 2 in, 1 out]
            n360 = call "Input_String_Dialog.vi"("Value"=w664, "Message to user"=w659) -> ("Ok Out"=w656:bool, "Output string"=w658:string)
            n361 = case shown="False" w656 {
              tunnel: w658 -> [_ w669]
              tunnel: [w665 w668] -> w657
              frame False {
                n362 = property on="Default Traverse Name" class="Ring (strict)"() -> ("Strings []"=w666:string[])  [unwired: 2 in, 2 out]
                n363 = Index Array(array=w666, index=0) -> (element=w665:string)
              }
              frame True {
                n364 = call "Fast_string_Replace.vi"("Replace match with:"="_", "Input String"=w669, "regular expression"=" ") -> ("Output String"=w668:string)  [unwired: 2 out]
              }
            }
          }
          frame True {
          }
        }
        n365 = global write "Trav_pos_global.vi" "Default Traverse Setup"(w647) -> ()
      }
      frame "Update Traverse setup menu ring" {
        n366 = global read "Trav_pos_global.vi" "Default Traverse Setup"() -> (w677:string)
        n367 = local read "Data Folder"() -> (w683:path)
        n368 = Build Path(base path=w683, name or relative path="Preferences") -> (appended path=w682:path)
        n369 = Build Path(base path=w682, name or relative path=w675) -> (appended path=w681:path)
        n370 = List Folder(path=w681) -> (folder names=w679:string[])  [unwired: 1 in, 5 out]
        n371 = Build Array (concatenate)(w679, "--New Traverse Setup--") -> (w678:string[])
        n372 = Search 1D Array(1D array=w678, element=w677) -> (index of element=w685:i32)  [unwired: 1 out]
        n373 = case shown="-1" w685 {
          tunnel: [w691 0] -> w687
          tunnel: w678 -> [w690 w694]
          tunnel: w677 -> [_ w693]
          tunnel: w685 -> [w691 _]
          tunnel: [w690 w692] -> w676
          frame 0, Default {
          }
          frame -1 {
            n374 = Build Array (concatenate)(w693, w694) -> (w692:string[])
          }
        }
        n375 = local write "Default Traverse Name"(w687) -> ()
        n376 = property on="Default Traverse Name" class="Ring (strict)"("Strings []"=w676) -> ()  [unwired: 2 in, 2 out]
      }
      frame "Create Traverse setup" {
        n377 = local read "Templates"() -> (w697:path)
        n378 = Build Path(base path=w697, name or relative path="All_Traverses") -> (appended path=w703:path)
        n379 = stacked-sequence {
          seq-local: [w708 _] -> [_ w736]
          seq-local: [w707 _] -> [_ _]
          tunnel: w703 -> [w710 _]
          tunnel: [w713 _] -> w700
          tunnel: [w712 _] -> w699
          tunnel: w697 -> [_ w735]
          tunnel: [_ w733] -> w696
          frame #0 {
            w716 = "Default_Space_file.xls" ("name or relative path")
            w711 = "Traverse_Setup.xls" ("name or relative path")
            n380 = global read "Trav_pos_global.vi" "Default Traverse Setup"() -> (w707:string)
            n381 = global read "Constants_global.vi" "Traverse folder"() -> (w720:path)
            n382 = Build Path(base path=w710, name or relative path=w716) -> (appended path=w714:path)
            n383 = Build Path(base path=w710, name or relative path=w711) -> (appended path=w709:path)
            n384 = Build Path(base path=w720, name or relative path=w707) -> (appended path=w708:path)
            n385 = Build Path(base path=w708, name or relative path="Trav_Space_Files") -> (appended path=w717:path)
            n386 = Build Path(base path=w717, name or relative path=w716) -> (appended path=w713:path)
            n387 = call "Does_file_exist_(simple).vi"("Pathname"=w713) -> ("exists?"=w715:bool)
            n388 = case shown="False" w715 {
              tunnel: w714 -> [w723 _]
              tunnel: w713 -> [w722 _]
              frame False {
                n389 = call "Create_directory_path.vi"("Path name"=w722) -> ("Path name Out"=w721:path)  [unwired: 1 in, 1 out]
                n390 = Copy(10:w721, 11:w723) -> ()  [unwired: 1 in, 5 out]
              }
              frame True {
              }
            }
            n391 = Build Path(base path=w708, name or relative path=w711) -> (appended path=w712:path)
            n392 = call "Does_file_exist_(simple).vi"("Pathname"=w712) -> ("exists?"=w719:bool)
            n393 = case shown="False" w719 {
              tunnel: w709 -> [w732 _]
              tunnel: w712 -> [w728 _]
              tunnel: w707 -> [w731 _]
              frame False {
                w724 = TRUE  # append to file? (new file:F)
                n394 = call "Create_directory_path.vi"("Path name"=w728) -> ("Path name Out"=w727:path)  [unwired: 1 in, 1 out]
                n395 = call "Read_File_Simple.vi"("Filename"=w732) -> ("string"=w730:string)  [unwired: 2 in, 7 out]
                n396 = call "Fast_string_Replace.vi"("Replace match with:"=w731, "Input String"=w730, "regular expression"="A_Tunnel") -> ("Output String"=w726:string)  [unwired: 2 out]
                n397 = call "Write_Characters_To_File.vi"("file path (dialog if empty)"=w727, "advisory dialog? (display:T)"=TRUE, "character string"=w726, "append to file? (new file:F)"=w724) -> ()  [unwired: 1 in, 4 out]
              }
              frame True {
              }
            }
          }
          frame #1 {
            w734 = "Traverse_Preferences.txt" ("name or relative path")
            n398 = Build Path(base path=w736, name or relative path=w734) -> (appended path=w733:path)
            n399 = Build Path(base path=w735, name or relative path=w734) -> (appended path=w737:path)
            n400 = call "Does_file_exist_(simple).vi"("Pathname"=w733) -> ("exists?"=w738:bool)
            n401 = case shown="False" w738 {
              tunnel: w737 -> [w741 _]
              tunnel: w733 -> [w740 _]
              frame False {
                n402 = call "Create_directory_path.vi"("Path name"=w740) -> ("Path name Out"=w739:path)  [unwired: 1 in, 1 out]
                n403 = Copy(10:w739, 11:w741) -> ()  [unwired: 1 in, 5 out]
              }
              frame True {
              }
            }
          }
        }
        n404 = Build Array (concatenate)(w702, w699, w696, w700) -> (w701:path[])
      }
      frame "Check file permission status" {
        n405 = local read "Post Processing Machine"() -> (w742:bool)
        n406 = for {
          tunnel: w747 -> [w761] mode=indexing
          shift-right: [w758] -> w744
          shift-left: "" -> [w759]
          n407 = call "Can_File_be_Editted.vi"("Filename"=w761) -> ("File Permissions OK?"=w762:bool, "Comment String"=w760:string)  [unwired: 2 out]
          n408 = case shown="False" w762 {
            tunnel: w761 -> [w767 _]
            tunnel: w760 -> [w766 _]
            tunnel: w759 -> [w765 w768]
            tunnel: [w764 w768] -> w758
            frame False {
              n409 = Format Into String(format string="\"%s\" %s\n", initial string=w765, w767, w766) -> (resulting string=w764:string)  [unwired: 1 in, 1 out]
            }
            frame True {
            }
          }
        }
        n410 = case shown="\"Load, Edit then Save\"" w748 {
          tunnel: [w770 w774] -> w749
          tunnel: w742 -> [w769 w773]
          frame "Save Preferences to file", Default {
            n411 = Select(t="Save Preference File", s=w769, f="Output Dev Number") -> (s? t:f=w770:string)
          }
          frame "Load, Edit then Save" {
            n412 = Select(t="Data Folder Changed?", s=w773, f="What next1") -> (s? t:f=w774:string)
          }
        }
        n413 = Empty String/Path?(string/path=w744) -> (empty?=w745:bool)
        n414 = case shown="True" w745 {
          tunnel: w744 -> [w757 _]
          frame False {
            n415 = Concatenate Strings("The following file permissions need to be sorted out before the software will run correctly.\n\n" ("string"), w757) -> (w755:string)
            n416 = Two Button Dialog(message=w755, 1:"Continue" ("F button name (\"Cancel\")"), 2:"Abort" ("F button name (\"Cancel\")")) -> (T button?=w752:bool)
            n417 = Stop(stop? (T)=w752) -> ()
          }
          frame True {
          }
        }
      }
      frame "What next1" {
        n418 = property on="Rig Setup" class="Ring (strict)"() -> ("Strings []"=w779:string[])  [unwired: 2 in, 2 out]
        n419 = Array Size(array=w779) -> (size(s)=w783:i32)
        n420 = Decrement(x=w783) -> (x-1=w782:i32)
        n421 = Equal?(x=w782, y="Rig Setup") -> (x = y?=w781:bool)
        n422 = case shown="False" w781 {
          tunnel: [w787 "Please Enter New Rig Name" ("t")] -> w780
          tunnel: w779 -> [w790 _]
          tunnel: "Rig Setup" -> [w789 _]
          frame False {
            n423 = global read "Preference_global.vi" "Rig Setup"() -> (w791:string)
            n424 = Index Array(array=w790, index=w789) -> (element=w786:string)
            n425 = Not Equal?(x=w786, y=w791) -> (x != y?=w788:bool)
            n426 = case shown="False" w788 {
              tunnel: ["What next2" ("f") "Update Rig setup menu ring" ("t")] -> w787
              tunnel: w786 -> [_ w793]
              frame False {
              }
              frame True {
                n427 = global write "Preference_global.vi" "Rig Setup"(w793) -> ()
              }
            }
          }
          frame True {
            n428 = global write "Preference_global.vi" "Rig Setup"("") -> ()
          }
        }
      }
      frame "What next2" {
        n429 = property on="Default Traverse Name" class="Ring (strict)"() -> ("Strings []"=w799:string[])  [unwired: 2 in, 2 out]
        n430 = Array Size(array=w799) -> (size(s)=w803:i32)
        n431 = Decrement(x=w803) -> (x-1=w802:i32)
        n432 = Equal?(x=w802, y="Default Traverse Name") -> (x = y?=w801:bool)
        n433 = case shown="False" w801 {
          tunnel: [w807 "Please Enter new  Traverse Setup" ("t")] -> w800
          tunnel: w799 -> [w811 _]
          tunnel: "Default Traverse Name" -> [w810 _]
          frame False {
            n434 = global read "Trav_pos_global.vi" "Default Traverse Setup"() -> (w809:string)
            n435 = Index Array(array=w811, index=w810) -> (element=w806:string)
            n436 = Not Equal?(x=w806, y=w809) -> (x != y?=w808:bool)
            n437 = case shown="False" w808 {
              tunnel: ["Data Folder Changed?" ("f") "Update Traverse setup menu ring" ("t")] -> w807
              tunnel: w806 -> [_ w813]
              frame False {
              }
              frame True {
                n438 = global write "Trav_pos_global.vi" "Default Traverse Setup"(w813) -> ()
              }
            }
          }
          frame True {
            n439 = global write "Trav_pos_global.vi" "Default Traverse Setup"("") -> ()
          }
        }
      }
      frame "Data Folder Changed?" {
        w819 = "Please Select your data folder"
        n440 = global read "Constants_global.vi" "Data Folder"() -> (w825:path)
        n441 = local read "Data Folder"() -> (w826:path)
        n442 = property on="OK" class="Bool (strict)"("Visible"=TRUE) -> ()  [unwired: 2 in, 2 out]
        n443 = while {
          shift-right: [w835] -> _
          shift-left: _ -> [w834]
          tunnel: [w833] -> w821
          stop <- TRUE stop-if-true
          n444 = local read "Post Processing Machine"() -> (w835:bool)
          n445 = Not Equal?(x=w835, y=w834) -> (x != y?=w833:bool)
        }
        n446 = Not Equal?(x=w825, y=w826) -> (x != y?=w817:bool)
        n447 = Select(t=w819, s=w817, f="Has OK has been pressed?") -> (s? t:f=w818:string)
        n448 = case shown="True" w821 {
          tunnel: [w829 w831] -> w820
          tunnel: w819 -> [_ w831]
          tunnel: w818 -> [w829 _]
          frame False {
          }
          frame True {
            n449 = global write "Preference_global.vi" "Rig Setup"("") -> ()
          }
        }
      }
      frame "Has OK has been pressed?" {
        n450 = flat-sequence {
          tunnel: ["OK"] -> w837
          frame #0 {
            n451 = Wait (ms)(milliseconds to wait=u32 100) -> ()  [unwired: 1 out]
          }
          frame #1 {
          }
        }
        n452 = local read "Post Processing Machine"() -> (w838:bool)
        n453 = case shown="True" w837 {
          tunnel: w838 -> [w843 w849]
          tunnel: [w842 w846] -> w836
          frame False {
            n454 = Select(t="Data Folder Changed?", s=w843, f="What next1") -> (s? t:f=w842:string)
          }
          frame True {
            n455 = Select(t="Save Preference File", s=w849, f="Output Dev Number") -> (s? t:f=w846:string)
          }
        }
      }
      frame "Output Dev Number" {
        n456 = stacked-sequence {
          seq-local: [w857 _ _] -> [_ w893 _]
          tunnel: w854 -> [_ _ _]
          frame #0 {
            w860 = T12 0 items=["Canonical Names Only"=0, "Aliases Only"=1, "Include Matching Aliases"=2, "Include All Aliases"=4] ("Search Mode")
            n457 = VISA Find Resource(10:w860) -> (3:w859:string[])  [unwired: 1 in, 3 out]
            n458 = for {
              shift-right: [w875] -> w857
              shift-left: string[] [] -> [w876]
              tunnel: w859 -> [w865] mode=indexing
              n459 = Reverse String(1:w865) -> (0:w873:string)
              n460 = Match Pattern(string=w873, regular expression="::") -> (before substring=w872:string)  [unwired: 4 out]
              n461 = Match Pattern(string=w865, regular expression="NI-VISA") -> (offset past match=w864:i32)  [unwired: 4 out]
              n462 = Reverse String(1:w872) -> (0:w870:string)
              n463 = Less Than 0?(x=w864) -> (x < 0?=w862:bool)
              n464 = Equal?(x=w870, y="INSTR") -> (x = y?=w868:bool)
              n465 = Equal?(x=w870, y="RAW") -> (x = y?=w867:bool)
              n466 = Or(x=w868, y=w867) -> (x .or. y?=w863:bool)
              n467 = And(x=w863, y=w862) -> (x .and. y?=w861:bool)
              n468 = case shown="True" w861 {
                tunnel: w876 -> [w877 w880]
                tunnel: [w877 w879] -> w875
                tunnel: w865 -> [_ w878]
                frame False {
                }
                frame True {
                  n469 = Build Array (concatenate)(w880, w878) -> (w879:string[])
                }
              }
            }
          }
          frame #1 {
            w885 = "Dev" ("format string")
            n470 = local read "Analogue Device Serial No."() -> (w889:string)
            n471 = String Length(string=w885) -> (length=w887:i32)
            n472 = local read "PWA Device Serial No."() -> (w883:string)
            n473 = String Subset(string=w889, length (rest)=w887) -> (substring=w891:string)  [unwired: 1 out]
            n474 = String Subset(string=w883, length (rest)=w887) -> (substring=w886:string)  [unwired: 1 out]
            n475 = Equal?(x=w891, y=w885) -> (x = y?=w888:bool)
            n476 = Equal?(x=w885, y=w886) -> (x = y?=w884:bool)
            n477 = for {
              tunnel: w889 -> [w912]
              tunnel: w893 -> [w910] mode=indexing
              tunnel: [w911] -> w905 mode=indexing
              tunnel: w883 -> [w909]
              tunnel: [w908] -> w902 mode=indexing
              n478 = Match Pattern(string=w910, regular expression=w912) -> (offset past match=w911:i32)  [unwired: 1 in, 3 out]
              n479 = Match Pattern(string=w910, regular expression=w909) -> (offset past match=w908:i32)  [unwired: 1 in, 3 out]
            }
            n480 = Array Max & Min(array=w905) -> (max index (indices)=w906:i32)  [unwired: 3 out]
            n481 = Array Max & Min(array=w902) -> (max index (indices)=w904:i32)  [unwired: 3 out]
            n482 = Increment(x=w904) -> (x+1=w895:i32)
            n483 = Increment(x=w906) -> (x+1=w899:i32)
            n484 = Equal To 0?(x=w899) -> (x = 0?=w901:bool)
            n485 = Equal To 0?(x=w895) -> (x = 0?=w896:bool)
            n486 = Select(t=1, s=w901, f=w899) -> (s? t:f=w900:i32)
            n487 = Select(t=1, s=w896, f=w895) -> (s? t:f=w894:i32)
            n488 = Format Into String(format string="Dev%d", w900) -> (resulting string=w890:string)  [unwired: 2 in, 1 out]
            n489 = Format Into String(format string="Dev%d", w894) -> (resulting string=w882:string)  [unwired: 2 in, 1 out]
            n490 = Select(t=w889, s=w888, f=w890) -> (s? t:f=w892:string)
            n491 = Select(t=w883, s=w884, f=w882) -> (s? t:f=w881:string)
            n492 = global write "PWAtasksGLOBAL.vi" "Analogue Dev Name"(w892) -> ()
            n493 = global write "PWAtasksGLOBAL.vi" "PWA Dev Name"(w881) -> ()
          }
          frame #2 {
            n494 = for {
              tunnel: string[] ["Raw_Calibrations", "Raw_Measurements", "Results", "Calibrations", "Commands"] -> [w917] mode=indexing
              n495 = call "Data_folder_Path.vi"("Data Type"=w917) -> ("Data Folder"=w916:path)  [unwired: 4 in]
              n496 = Build Path(base path=w916, name or relative path="Test" ("Substring")) -> (appended path=w919:path)
              n497 = call "Create_directory_path.vi"("Path name"=w919) -> ()  [unwired: 1 in, 2 out]
            }
            n498 = call "Data_folder_Path.vi"("Data Type"="Results_Post_Processed" ("element")) -> ("Data Folder"=w913:path)  [unwired: 4 in]
            n499 = call "Create_directory_path.vi"("Path name"=w913) -> ()  [unwired: 1 in, 2 out]
          }
        }
      }
      frame "Save Preference File" {
        n500 = call "Date_and_Time_to_string.vi"() -> ("Date and time (spreadsheet)"=w931:string)
        n501 = call "Setup_Filepath.vi"("Setup File Type"=Setup_Filetype."General", "Filename in"=w921) -> ("Filename Out"=w920:path)  [unwired: 1 out]
        n502 = for {
          tunnel: w930 -> [w941] mode=indexing
          shift-right: [w937] -> w929
          shift-left: w931 -> [w939]
          n503 = case shown="\"Traverse to Traverse Collision Detection\"" w941 {
            tunnel: w941 -> [w944 _ _ _ _ _ _ _ _ _ _ _ _ _ _ _ _ _ _ _]
            tunnel: ["No Match" "Server address" "EnFlo_Data_Folder_Setup" w948 w950 w952 w956 w960 "SMTP server IP address" "PWA Device Serial No." "Analogue Device Serial No." w965 w966 w968 "Temperature" "Abs Press (mbar)" w973 w978 w981 w984] -> w940
            frame "No Match", Default {
              n504 = call "Was_string_matched.vi"("Match Error"=TRUE, "Variable name"=w944) -> ()  [unwired: 1 in]
            }
            frame "Server address" {
              n505 = global write "Preference_global.vi" "Server address"("Server address") -> ()
            }
            frame "EnFlo_Data_Folder_Setup" {
              n506 = global write "Preference_global.vi" "EnFlo_Data_Folder_Setup"("EnFlo_Data_Folder_Setup") -> ()
            }
            frame "Server port number" {
              n507 = global write "Preference_global.vi" "Server port number"("Server port number") -> ()
              n508 = Number To Decimal String(number="Server port number") -> (decimal integer string=w948:string)  [unwired: 1 out]
            }
            frame "Default Source Establishment Time (s)" {
              n509 = global write "Preference_global.vi" "Default Source Establishment Time (s)"("Default Source Establishment Time (s)") -> ()
              n510 = Number To Decimal String(number="Default Source Establishment Time (s)") -> (decimal integer string=w950:string)  [unwired: 1 out]
            }
            frame "Tunnel Speed Control" {
              n511 = global write "Preference_global.vi" "Tunnel Speed Control"("Tunnel Speed Control") -> ()
              n512 = Select(t="TRUE", s="Tunnel Speed Control", f="FALSE") -> (s? t:f=w952:string)
            }
            frame "Traverse to Traverse Collision Detection" {
              n513 = global write "Preference_global.vi" "Traverse to Traverse Collision Detection"("Traverse to Traverse Collision Detection") -> ()
              n514 = Select(t="TRUE", s="Traverse to Traverse Collision Detection", f="FALSE") -> (s? t:f=w956:string)
            }
            frame "LabVIEW Administrators" {
              n515 = global write "Preference_global.vi" "LabVIEW Administrators"("LabVIEW Administrators") -> ()
              n516 = call "Put_Array_into_String.vi"("String array"="LabVIEW Administrators") -> ("String Value"=w960:string)
            }
            frame "SMTP server IP address" {
              n517 = global write "Preference_global.vi" "SMTP server IP address"("SMTP server IP address") -> ()
            }
            frame "PWA Device Serial No." {
            }
            frame "Analogue Device Serial No." {
            }
            frame "DataTranslation Device No." {
              n518 = global write "Preference_global.vi" "DataTranslation Device No."("DataTranslation Device No.") -> ()
              n519 = Number To Decimal String(number="DataTranslation Device No.") -> (decimal integer string=w965:string)  [unwired: 1 in]
            }
            frame "Default Traverse Name" {
              n520 = global read "Trav_pos_global.vi" "Default Traverse Setup"() -> (w966:string)
            }
            frame "Server Comms" {
              n521 = case shown="\"Server Link Healthy\"" "Server Comms" {
                tunnel: ["TRUE" "FALSE"] -> w968
                frame "Server Link Healthy" {
                }
                frame "Do Not Link To Server" {
                }
              }
              n522 = global write "Preference_global.vi" "Server Comms"("Server Comms") -> ()
            }
            frame "Temperature" {
              n523 = global write "Preference_global.vi" "Temperature"("Temperature") -> ()
            }
            frame "Abs Press (mbar)" {
              n524 = global write "Preference_global.vi" "Abs Press (mbar)"("Abs Press (mbar)") -> ()
            }
            frame "Current Overhead Factor" {
              n525 = call "Overhead_Factor.vi"("Mode"=Overhead."Read Current Overhead") -> ("Current Overhead Factor"=w975:dbl)  [unwired: 3 in]
              n526 = Number To Fractional String(number=w975, precision (6)=i16 4) -> (F-format string=w973:string)  [unwired: 2 out]
            }
            frame "Auto Calib Error fr Previous" {
              n527 = global write "Preference_global.vi" "% Error From Previous Calib"("% Error From Previous Calib") -> ()
              n528 = Number To Fractional String(number="% Error From Previous Calib", precision (6)=i16 2) -> (F-format string=w978:string)  [unwired: 2 out]
            }
            frame "Auto Calib Error fr First" {
              n529 = global write "Preference_global.vi" "% Error From First Calib"("% Error From First Calib") -> ()
              n530 = Number To Fractional String(number="% Error From First Calib", precision (6)=i16 2) -> (F-format string=w981:string)  [unwired: 2 out]
            }
            frame "EnFlo_Data_Central_Repository" {
              n531 = global read "Constants_global.vi" "EnFlo_Data_Central_Repository"() -> (w983:path)
              n532 = Path To String(path=w983) -> (string=w984:string)
            }
          }
          n533 = call "Characters_to_string.vi"("Characters to write"=w940, "Label for characters"=w941) -> ("Output string"=w938:string)
          n534 = Concatenate Strings(w939, w938) -> (w937:string)
        }
        n535 = case shown="\"Load, Edit then Save\"" w925 {
          tunnel: [TRUE TRUE TRUE] -> w924
          frame "Load, Edit then Save" {
            n536 = Current VI's Path() -> (path=w933:path)
            n537 = call "Open_Close_Front_Panel.ph.vi"("Front Panel Window:Open"=FALSE, "VI path"=w933) -> ()  [unwired: 2 out]
          }
          frame "Load Preferences from file" {
          }
          frame "Save Preferences to file" {
          }
        }
        n538 = call "Write_Characters_To_File.vi"("file path (dialog if empty)"=w920, "advisory dialog? (display:T)"=FALSE, "character string"=w929, "append to file? (new file:F)"=FALSE) -> ()  [unwired: 1 in, 4 out]
      }
      frame "Save SW Preferences" {
        w1004 = FALSE  # append to file? (new file:F)
        w1005 = FALSE  # advisory dialog? (display:T)
        n539 = local read "Post Processing Machine"() -> (w994:bool)
        n540 = global read "Preference_global.vi" "User_Name"() -> (w987:string)
        n541 = Path To String(path="Data Folder") -> (string=w996:string)
        n542 = global read "Preference_global.vi" "Server Comms"() -> (w1000:T3)
        n543 = call "Characters_to_string.vi"("Characters to write"=w996, "Label for characters"=w998) -> ("Output string"=w1006:string)
        n544 = Select(t="True", s=w994, f="False") -> (s? t:f=w991:string)
        n545 = call "Characters_to_string.vi"("Characters to write"=w987, "Label for characters"=w988) -> ("Output string"=w986:string)
        n546 = call "Characters_to_string.vi"("Characters to write"=w991, "Label for characters"=w989) -> ("Output string"=w990:string)
        n547 = call "Date_and_Time_to_string.vi"() -> ("Date and time (spreadsheet)"=w1001:string)
        n548 = case shown="\"Server Link Healthy\"" w1000 {
          tunnel: ["Update Served VI file" "Update Local Adam Table"] -> w999
          frame "Server Link Healthy" {
          }
          frame "Do Not Link To Server" {
          }
        }
        n549 = Concatenate Strings(w1001, w1006, w990, w986) -> (w1002:string)
        n550 = local read "EnFlo SW Preferences"() -> (w1003:path)
        n551 = call "Write_Characters_To_File.vi"("file path (dialog if empty)"=w1003, "advisory dialog? (display:T)"=w1005, "character string"=w1002, "append to file? (new file:F)"=w1004) -> ()  [unwired: 1 in, 4 out]
        n552 = case shown="True" "Reset Email Counter" {
          tunnel: "Reset Email Counter" -> [_ w1009]
          frame False {
          }
          frame True {
            n553 = global write "Preference_global.vi" "Unblock Email"(w1009) -> ()
          }
        }
      }
      frame "Update Local Adam Table" {
        n554 = stacked-sequence {
          seq-local: [w1021 _] -> [_ w1035]
          tunnel: ["Update Served VI file" _] -> w1013
          frame #0 {
            w1021 = T13 {"Ch Name"="", "Type"="", "Function"=enum."Analogue Input", "Ch State"=enum."On", "Calibration type"=enum."Raw", "A"=0.0, "B"=0.0, "C"=0.0, "D"=0.0, "Comments"="", "Address"={"Main"=0, "Ch."=0, "Sub"=0, "Port Name"=""}, "String"="", "Duty"=0} ("Ch Discription")
            n555 = global read "Preference_global.vi" "Abs Press (mbar)"() -> (w1018:string)
            n556 = global read "Preference_global.vi" "Temperature"() -> (w1019:string)
            n557 = Bundle By Name(cluster=w1021, "Type"=T9 "", "Calibration type"=Calib_type_ADAM."Raw", "A"=1.0) -> (w1022:T13)
            n558 = Build Array(w1019, w1018) -> (w1017:string[])
            n559 = for {
              tunnel: [w1028] -> w1020 mode=indexing
              tunnel: w1022 -> [w1027]
              tunnel: w1017 -> [w1026] mode=indexing
              n560 = Bundle By Name(cluster=w1027, "Ch Name"=w1026) -> (w1028:T13)
            }
            n561 = call "Update_Ch_Discription_client.vi"("Channels to update In"=w1020) -> ()  [unwired: 1 out]
          }
          frame #1 {
            n562 = global read "Preference_global.vi" "Rig Setup"() -> (w1030:string)
            n563 = call "Get_Current_Scan_client.vi"() -> ("Ch Description Array"=w1036:T13[])  [unwired: 1 in, 3 out]
            n564 = Match Pattern(string=w1030, regular expression="-") -> (before substring=w1029:string)  [unwired: 4 out]
            n565 = Format Into String(format string="%s Metadata:" ("Format String"), w1029) -> (resulting string=w1038:string)  [unwired: 2 in, 1 out]
            n566 = Initialize Array(w1035, 0 ("dimension size")) -> (w1033:T13[])
            n567 = for {
              shift-right: [w1049] -> w1032
              shift-left: w1033 -> [w1050]
              tunnel: w1036 -> [w1041] mode=indexing
              tunnel: w1038 -> [w1048]
              tunnel: "Metadata:" ("Format String") -> [w1047]
              n568 = Unbundle By Name(w1041) -> ("Ch Name"=w1040:string)
              n569 = Match Pattern(string=w1040, regular expression=w1048) -> (offset past match=w1045:i32)  [unwired: 4 out]
              n570 = Match Pattern(string=w1040, regular expression=w1047) -> (offset past match=w1046:i32)  [unwired: 4 out]
              n571 = Greater Or Equal To 0?(x=w1046) -> (x >= 0?=w1043:bool)
              n572 = Less Than 0?(x=w1045) -> (x < 0?=w1044:bool)
              n573 = And(x=w1044, y=w1043) -> (x .and. y?=w1042:bool)
              n574 = case shown="True" w1042 {
                tunnel: w1050 -> [w1051 w1056]
                tunnel: [w1051 w1055] -> w1049
                tunnel: w1041 -> [_ w1054]
                frame False {
                }
                frame True {
                  n575 = Bundle By Name(cluster=w1054, "Ch State"=Channel_State."Off") -> (w1052:T13)
                  n576 = Build Array (concatenate)(w1056, w1052) -> (w1055:T13[])
                }
              }
            }
            n577 = call "Update_Ch_Discription_client.vi"("Channels to update In"=w1032) -> ()  [unwired: 1 out]
          }
        }
      }
      frame "Update Served VI file" {
        # "Template"
        # "Orig"
        n578 = call "Setup_Filepath.vi"("Setup File Type"=Setup_Filetype."General", "Filename in"=w1058) -> ("Filename Out"=w1057:path)  [unwired: 1 out]
        n579 = Build Array("Served:VI:Name", "Served:VI:Path", "Server:IP Number:& Port No") -> (w1063:string[])
        n580 = stacked-sequence {
          seq-local: [w1068 _ _ _] -> [_ _ w1078 _]
          seq-local: [_ w1075 _ _] -> [_ _ w1079 _]
          seq-local: [_ _ w1080 _] -> [_ _ _ w1105]
          tunnel: w1063 -> [w1070 w1076 _ w1106]
          tunnel: w1057 -> [w1069 _ _ w1107]
          tunnel: w1058 -> [_ w1072 _ _]
          frame #0 {
            n581 = call "Read_Ch_data_file.vi"("Present Channels"=w1070, "Output"=enum16{"All Ch data", "The last few rows"}."All Ch data", "Filename"=w1069) -> ("Channel Values"=w1068:string[][])  [unwired: 2 in, 4 out]
          }
          frame #1 {
            n582 = local read "Templates"() -> (w1074:path)
            n583 = Build Path(base path=w1074, name or relative path=w1072) -> (appended path=w1073:path)
            n584 = call "Read_Ch_data_file.vi"("Present Channels"=w1076, "Output"=enum16{"All Ch data", "The last few rows"}."All Ch data", "Filename"=w1073) -> ("Channel Values"=w1075:string[][])  [unwired: 2 in, 4 out]
          }
          frame #2 {
            n585 = Index Array(array=w1078, index (col)=0 ("Index")) -> (element=w1083:string[])  [unwired: 1 in]
            n586 = To Upper Case(1:w1079) -> (0:w1081:string[][])
            n587 = To Upper Case(1:w1083) -> (0:w1082:string[])
            n588 = for {
              tunnel: w1082 -> [w1086]
              tunnel: w1079 -> [w1091] mode=indexing
              tunnel: w1081 -> [w1085] mode=indexing
              tunnel: [w1088] -> w1080 mode=indexing
              tunnel: w1078 -> [w1087]
              n589 = Index Array(array=w1085, index=0 ("Index")) -> (element=w1089:string)
              n590 = Search 1D Array(1D array=w1086, element=w1089) -> (index of element=w1090:i32)  [unwired: 1 out]
              n591 = case shown="0, Default" w1090 {
                tunnel: w1091 -> [w1100 w1101]
                tunnel: w1090 -> [w1097 _]
                tunnel: [w1093 w1101] -> w1088
                tunnel: w1087 -> [w1098 _]
                frame 0, Default {
                  n592 = Index Array(array=w1098, index (row)=w1097, index (col)=2 ("Index")) -> (element=w1095:string)
                  n593 = Array Subset(array=w1100, length=2) -> (w1094:string[])  [unwired: 1 in]
                  n594 = Build Array (concatenate)(w1094, w1095) -> (w1093:string[])
                }
                frame -1 {
                }
              }
            }
          }
          frame #3 {
            w1102 = FALSE  # Append last row only
            w1103 = FALSE  # Lock File
            w1104 = FALSE  # exists?
            n595 = call "Write_Ch_data_file.vi"("Append last row only"=w1102, "Lock File"=w1103, "exists?"=w1104, "Channel Values"=w1105, "Channel names"=w1106, "Filename"=w1107) -> ()  [unwired: 2 in, 4 out]
          }
        }
      }
      frame "Initialise Globals" {
        w1112 = TRUE  # OK
        w1116 = FALSE  # append to file? (new file:F)
        w1115 = FALSE  # advisory dialog? (display:T)
        n596 = global read "Constants_global.vi" "ADAM setups folder"() -> (w1122:path)
        n597 = global read "Constants_global.vi" "All_Users"() -> (w1111:path)
        n598 = property on="ADAM Setup File" class="Ring (strict)"() -> ("Strings []"=w1117:string[])  [unwired: 2 in, 2 out]
        n599 = Build Path(base path=w1111, name or relative path="Current_Username") -> (appended path=w1109:path)
        n600 = Build Path(base path=w1122, name or relative path="Setup_Files") -> (appended path=w1120:path)
        n601 = global read "Preference_global.vi" "User_Name"() -> (w1108:string)
        n602 = Build Path(base path=w1120, name or relative path="Selected_Filename.txt" ("Substring")) -> (appended path=w1113:path)
        n603 = call "Get_users_email_addresses.vi"("OK"=w1112) -> ()  [unwired: 5 out]
        n604 = Index Array(array=w1117, index="ADAM Setup File") -> (element=w1114:string)
        n605 = call "Write_File_Simple.vi"("character string"=w1108, "file path"=w1109) -> ()  [unwired: 1 in, 2 out]
        n606 = call "Write_Characters_To_File.vi"("file path (dialog if empty)"=w1113, "advisory dialog? (display:T)"=w1115, "character string"=w1114, "append to file? (new file:F)"=w1116) -> ()  [unwired: 1 in, 4 out]
      }
    }
  }
  n607 = call "Get_IP_Number.vi"() -> ("IP Number"=→"This Machine's IP Number":string)
